vi "220225-VNA RP FLAT.vi"() -> ()   [LabVIEW 2021]
uses:
  Channel parameters.ctl
  Spectrum data.ctl
  vna settings.ctl
  Resonnance detection.ctl
  b7fd31b3-4c8f-4ae8-a038-7c142e2eb182.vi
  <vilib>/Analysis/baseanly.llb/Mean (DBL).vi
  <vilib>/Utility/file.llb/Write Delimited Spreadsheet (DBL).vi
  <vilib>/Comparison/Equal/Equal Functor/Equal Functor.lvclass
  <vilib>/Analysis/NI_AALBase.lvlib
panel:
  in  "RP VNA SETTING":T1={"F start"=200000, "F stop"=2000500, "Sweep size"=1000, "Decimation"=5000, "F_corr"=0, "Ph_OUT1"=0, "Ph_OUT2"=0, "OUT_Lvl1"=32700, "OUT_Lvl2"=32700, "GPIO"=0}
  in  "Amplitude(1V)":dbl=0.3 format="%#_13g"
  out "RP CONNECT":bool
  in  "VOA Calibration cluster":cluster{"PUMP":dbl[], "PROBE":dbl[]}
  out "TRACK DATA REL NO SMOOTHING":dbl[][](array[numeric])
  out "TRACK DATA ABS NO SMOOTHING":dbl[][](array[numeric])
  in  "BTN SAVE TRACK":bool
  in  "BTN STOP TRACK":bool
  out "TRACK REPOSITERY":path
  out "TRACK DATA REL":dbl[][](array[numeric])
  out "TRACK DATA ABS":dbl[][](array[numeric])
  out "Track File List":path[](array[path])
  out "Track Repositery List":path[](array[path])
  out "CHANNEL CHOSEN":i32
  in  "TRACK-STOP":bool
  out "STATUS":string="STOP"
  out "track data":dbl[](array[numeric])=[495490.5081042979, 495481.56129759253, 495478.2328599854, 495479.84884744807, 495476.377462383, 495478.7819904735]
  out "MAIN TAB":T2(tab)
  out "ACQ Indicator":bool
  in  "PUMP":dbl(slide)=100.0 min=0.0 max=100.0 step=0.1 scale=0.0..100.0
  in  "PROBE":dbl(slide)=100.0 min=0.0 max=100.0 step=0.1 scale=0.0..100.0
  in  "BTN RESET VNA":bool
  in  "SPAN":dbl=1900.0 format="%#5.1f"
  in  "STOP":dbl=2000.0 format="%#5.1f"
  in  "CENTER":dbl=1050.0 format="%#5.1f"
  in  "BTN AF VNA":bool
  out "MAGNITUDE/PHASE":cluster{cluster{dbl, dbl}[]}[](graph)
  in  "CHANNEL CHOICE VNA":T3(radio)
  in  "BTN Center to max":bool
  in  "BTN ZOOM-":bool
  in  "BTN ZOOM+":bool
  in  "START":dbl=200.0 format="%#5.1f"
  out "SPACING":dbl=1900.0 min=0.0 max=100.0 step=0.5 format="%#5.1f"
  in  "Points N°":i32=1000 min=600 max=5000 step=1 format="%#4.4g"
  in  "BTN LOOP VNA":bool
  in  "BTN RUN VNA":bool
  in  "BTN SAVE VNA":bool
  in  "BTN FIT DISPLAY":bool caption="FIT DISPLAY"
  in  "BTN AUTOSCALE":bool caption="AUTOSCALE"
  in  "BTN DISPLAY TYPE":bool caption="DISPLAY"
  in  "BTN VIEW PERSISTANCE":bool
  in  "Hide/Show track data channel":bool[](array[boolean])
  in  "BTN AUTOSAVE RAW DATA":bool=TRUE
  in  "COMMENTS":string
  in  "ASSAY NAME":string
  in  "DELAY AFTER SWITCH (s)":i32
  in  "N°POINTS TO DISPLAY":i32=200
  in  "DISPLAY OPTION":u16(ring) items=["Absolute frequency", "Relative frequency (ppm)"]
  in  "DELAY BETWEEN TRIG (s)":i32
  in  "AVERAGE/POINT":dbl=1.0
  out "LIVE TRACK":dbl[][](graph)
  out "CHANNELS IND TRACK":T3(radio)
  in  "BTN RUN TRACK":bool
  in  "TEMPORAL SMOOTHING":i32=15
  in  "BTN NEW TRACK":bool
  in  "BTN PAUSE TRACK":bool
  in  "CHANNELS PARAMETERS":T4[](array[typedef])=[{"START 2"=200.0, "STOP 2"=2000.5, "CENTER 2"=1050.0, "SPAN 2"=1800.0, "CHANNEL TRACK ?"=FALSE, "PUMP"=100.0, "PROBE"=100.0, "Points N° 2"=1000, "SPACING 2"=100.0}, {"START 2"=200.0, "STOP 2"=2000.0, "CENTER 2"=1100.0, "SPAN 2"=1800.0, "CHANNEL TRACK ?"=FALSE, "PUMP"=100.0, "PROBE"=100.0, "Points N° 2"=1000, "SPACING 2"=1800.0}, {"START 2"=200.0, "STOP 2"=2000.0, "CENTER 2"=1100.0, "SPAN 2"=1800.0, "CHANNEL TRACK ?"=FALSE, "PUMP"=100.0, "PROBE"=100.0, "Points N° 2"=1000, "SPACING 2"=1800.0}, {"START 2"=200.0, "STOP 2"=2000.0, "CENTER 2"=1100.0, "SPAN 2"=1800.0, "CHANNEL TRACK ?"=FALSE, "PUMP"=100.0, "PROBE"=100.0, "Points N° 2"=1000, "SPACING 2"=1800.0}, {"START 2"=200.0, "STOP 2"=2000.0, "CENTER 2"=1100.0, "SPAN 2"=1800.0, "CHANNEL TRACK ?"=FALSE, "PUMP"=100.0, "PROBE"=100.0, "Points N° 2"=1000, "SPACING 2"=1800.0}, {"START 2"=200.0, "STOP 2"=2000.0, "CENTER 2"=1100.0, "SPAN 2"=1800.0, "CHANNEL TRACK ?"=FALSE, "PUMP"=100.0, "PROBE"=100.0, "Points N° 2"=1000, "SPACING 2"=1800.0}, {"START 2"=200.0, "STOP 2"=2000.0, "CENTER 2"=1100.0, "SPAN 2"=1800.0, "CHANNEL TRACK ?"=FALSE, "PUMP"=100.0, "PROBE"=100.0, "Points N° 2"=1000, "SPACING 2"=1800.0}, {"START 2"=200.0, "STOP 2"=2000.0, "CENTER 2"=1100.0, "SPAN 2"=1800.0, "CHANNEL TRACK ?"=FALSE, "PUMP"=100.0, "PROBE"=100.0, "Points N° 2"=1000, "SPACING 2"=1800.0}, {"START 2"=200.0, "STOP 2"=2000.0, "CENTER 2"=1100.0, "SPAN 2"=1800.0, "CHANNEL TRACK ?"=FALSE, "PUMP"=100.0, "PROBE"=100.0, "Points N° 2"=1000, "SPACING 2"=1800.0}, {"START 2"=200.0, "STOP 2"=2000.0, "CENTER 2"=1100.0, "SPAN 2"=1800.0, "CHANNEL TRACK ?"=FALSE, "PUMP"=100.0, "PROBE"=100.0, "Points N° 2"=1000, "SPACING 2"=1800.0}, {"START 2"=200.0, "STOP 2"=2000.0, "CENTER 2"=1100.0, "SPAN 2"=1800.0, "CHANNEL TRACK ?"=FALSE, "PUMP"=100.0, "PROBE"=100.0, "Points N° 2"=1000, "SPACING 2"=1800.0}, {"START 2"=200.0, "STOP 2"=2000.0, "CENTER 2"=1100.0, "SPAN 2"=1800.0, "CHANNEL TRACK ?"=FALSE, "PUMP"=100.0, "PROBE"=100.0, "Points N° 2"=1000, "SPACING 2"=1800.0}, {"START 2"=200.0, "STOP 2"=2000.0, "CENTER 2"=1100.0, "SPAN 2"=1800.0, "CHANNEL TRACK ?"=FALSE, "PUMP"=100.0, "PROBE"=100.0, "Points N° 2"=1000, "SPACING 2"=1800.0}, {"START 2"=200.0, "STOP 2"=2000.0, "CENTER 2"=1100.0, "SPAN 2"=1800.0, "CHANNEL TRACK ?"=FALSE, "PUMP"=100.0, "PROBE"=100.0, "Points N° 2"=1000, "SPACING 2"=1800.0}, {"START 2"=200.0, "STOP 2"=2000.0, "CENTER 2"=1100.0, "SPAN 2"=1800.0, "CHANNEL TRACK ?"=FALSE, "PUMP"=100.0, "PROBE"=100.0, "Points N° 2"=1000, "SPACING 2"=1800.0}, {"START 2"=200.0, "STOP 2"=2000.0, "CENTER 2"=1100.0, "SPAN 2"=1800.0, "CHANNEL TRACK ?"=FALSE, "PUMP"=100.0, "PROBE"=100.0, "Points N° 2"=1000, "SPACING 2"=1800.0}] {"SPACING 2" min=0.0 max=100.0 step=0.5; "Points N° 2" min=0 max=100 step=1; "PROBE" min=0.0 max=100.0 step=0.5; "PUMP" min=0.0 max=100.0 step=0.5}
  out "CHANNEL IND SETTINGS":T5(radio)
  in  "RESONNANCE DETECTION":T6={"METHOD"=0, "Parabolic fit"={"Span type"=0, "Fit span"=100.0}} {"Parabolic fit"."Span type" items=["Points N°", "Frequency (Hz)", "Span %"]; "METHOD" items=["Maximum amplitude", "Max on parabolic fit"]}
  in  "TRACK DATA PARAMETERS":cluster{"MAIN FOLDER":path}={"MAIN FOLDER"=path "C:/SensWay Data"}
  in  "SPECTRUM POST PROCESSING PARAMETERS":cluster{"N° SMOOTHING POINTS":i32}={"N° SMOOTHING POINTS"=50}
  in  "AUTOFOCUS PARAMETERS":cluster{"ITERATIONS":i32}={"ITERATIONS"=5}
  in  "CHANNELS":T7
  in  "NETWORK PARAMETERS":T8={"RP-IP 1"="192.168.0.3", "RP-IP 2"="192.168.0.4", "RP-MAC 1"="", "RP-MAC 2"=""}
  in  "VNA DATA CLUSTER":T9
  in  "TRACK DATA CLUSTER":cluster{"CHANNEL":dbl, "KPI 1 TRACK":ext[]}
  out "LOOP ACT":bool
  out "RAW Freq table":dbl[](array[numeric])=[200000.0, 201802.3023023023, 203604.6046046046, 205406.9069069069, 207209.20920920922, 209011.51151151152, 210813.81381381382, 212616.1161161161, 214418.4184184184, 216220.7207207207, 218023.02302302304, 219825.32532532534, 221627.62762762763, 223429.92992992993, 225232.23223223223, 227034.53453453453, 228836.83683683682, 230639.13913913915, 232441.44144144145, 234243.74374374375, 236046.04604604605, 237848.34834834834, 239650.65065065064, 241452.95295295294, 243255.25525525527, 245057.55755755756, 246859.85985985986, 248662.16216216216, 250464.46446446446, 252266.76676676676, 254069.06906906905, 255871.37137137138, 257673.67367367368, 259475.97597597598, 261278.27827827827, 263080.5805805806, 264882.8828828829, 266685.18518518517, 268487.4874874875, 270289.7897897898, 272092.0920920921, 273894.39439439436, 275696.6966966967, 277498.998998999, 279301.3013013013, 281103.6036036036, 282905.9059059059, 284708.2082082082, 286510.51051051053, 288312.8128128128, 290115.1151151151, 291917.4174174174, 293719.7197197197, 295522.02202202205, 297324.3243243243, 299126.6266266266, 300928.9289289289, 302731.23123123124, 304533.5335335335, 306335.83583583584, 308138.1381381381, 309940.44044044043, 311742.74274274276, 313545.04504504503, 315347.34734734736, 317149.6496496496, 318951.95195195195, 320754.2542542543, 322556.55655655655, 324358.8588588588, 326161.16116116114, 327963.4634634635, 329765.76576576574, 331568.06806806807, 333370.37037037034, 335172.67267267266, 336974.974974975, 338777.27727727726, 340579.5795795796, 342381.88188188185, 344184.1841841842, 345986.4864864865, 347788.7887887888, 349591.09109109105, 351393.3933933934, 353195.6956956957, 354997.997997998, 356800.3003003003, 358602.60260260256, 360404.9049049049, 362207.2072072072, 364009.50950950955, 365811.8118118118, 367614.1141141141, 369416.4164164164, 371218.71871871874, 373021.021021021, 374823.3233233233, 376625.6256256256, 378427.9279279279, 380230.23023023026, 382032.5325325325, 383834.8348348348, 385637.1371371371, 387439.43943943945, 389241.7417417418, 391044.04404404404, 392846.3463463463, 394648.64864864864, 396450.95095095097, 398253.25325325324, 400055.5555555555, 401857.85785785783, 403660.16016016016, 405462.4624624625, 407264.76476476475, 409067.067067067, 410869.36936936935, 412671.6716716717, 414473.973973974, 416276.2762762763, 418078.57857857854, 419880.88088088087, 421683.1831831832, 423485.48548548546, 425287.7877877878, 427090.09009009006, 428892.3923923924, 430694.6946946947, 432496.996996997, 434299.29929929925, 436101.6016016016, 437903.9039039039, 439706.20620620623, 441508.5085085085, 443310.81081081077, 445113.1131131131, 446915.4154154154, 448717.7177177177, 450520.02002002, 452322.3223223223, 454124.6246246246, 455926.92692692694, 457729.2292292292, 459531.5315315315, 461333.8338338338, 463136.13613613613, 464938.4384384384, 466740.74074074073, 468543.04304304306, 470345.3453453453, 472147.64764764765, 473949.9499499499, 475752.25225225225, 477554.5545545545, 479356.85685685684, 481159.1591591592, 482961.46146146144, 484763.76376376377, 486566.06606606604, 488368.36836836836, 490170.67067067063, 491972.97297297296, 493775.2752752753, 495577.57757757755, 497379.8798798799, 499182.18218218215, 500984.4844844845, 502786.78678678675, 504589.0890890891, 506391.3913913914, 508193.69369369367, 509995.995995996, 511798.29829829826, 513600.6006006006, 515402.90290290286, 517205.2052052052, 519007.5075075075, 520809.8098098098, 522612.1121121121, 524414.4144144144, 526216.7167167168, 528019.0190190191, 529821.3213213213, 531623.6236236236, 533425.9259259258, 535228.2282282282, 537030.5305305305, 538832.8328328328, 540635.1351351351, 542437.4374374375, 544239.7397397398, 546042.042042042, 547844.3443443443, 549646.6466466465, 551448.9489489489, 553251.2512512512, 555053.5535535535, 556855.8558558559, 558658.1581581582, 560460.4604604605, 562262.7627627627, 564065.065065065, 565867.3673673674, 567669.6696696696, 569471.9719719719, 571274.2742742742, 573076.5765765766, 574878.8788788789, 576681.1811811812, 578483.4834834835, 580285.7857857858, 582088.0880880881, 583890.3903903903, 585692.6926926926, 587494.994994995, 589297.2972972973, 591099.5995995996, 592901.9019019019, 594704.2042042043, 596506.5065065065, 598308.8088088088, 600111.111111111, 601913.4134134133, 603715.7157157157, 605518.018018018, 607320.3203203203, 609122.6226226226, 610924.924924925, 612727.2272272272, 614529.5295295295, 616331.8318318318, 618134.134134134, 619936.4364364364, 621738.7387387387, 623541.041041041, 625343.3433433434, 627145.6456456457, 628947.947947948, 630750.2502502502, 632552.5525525525, 634354.8548548548, 636157.1571571571, 637959.4594594594, 639761.7617617617, 641564.0640640641, 643366.3663663664, 645168.6686686687, 646970.9709709709, 648773.2732732733, 650575.5755755756, 652377.8778778778, 654180.1801801801, 655982.4824824824, 657784.7847847848, 659587.0870870871, 661389.3893893894, 663191.6916916918, 664993.993993994, 666796.2962962963, 668598.5985985985, 670400.9009009008, 672203.2032032032, 674005.5055055055, 675807.8078078078, 677610.1101101101, 679412.4124124125, 681214.7147147147, 683017.017017017, 684819.3193193192, 686621.6216216215, 688423.9239239239, 690226.2262262262, 692028.5285285285, 693830.8308308308, 695633.1331331332, 697435.4354354354, 699237.7377377377, 701040.04004004, 702842.3423423423, 704644.6446446446, 706446.9469469469, 708249.2492492492, 710051.5515515516, 711853.8538538539, 713656.1561561562, 715458.4584584584, 717260.7607607607, 719063.063063063, 720865.3653653653, 722667.6676676676, 724469.9699699699, 726272.2722722723, 728074.5745745746, 729876.8768768768, 731679.1791791791, 733481.4814814815, 735283.7837837838, 737086.0860860861, 738888.3883883883, 740690.6906906907, 742492.992992993, 744295.2952952953, 746097.5975975975, 747899.8998998998, 749702.2022022022, 751504.5045045045, 753306.8068068068, 755109.109109109, 756911.4114114114, 758713.7137137137, 760516.016016016, 762318.3183183183, 764120.6206206206, 765922.9229229229, 767725.2252252252, 769527.5275275275, 771329.8298298299, 773132.1321321321, 774934.4344344344, 776736.7367367367, 778539.039039039, 780341.3413413413, 782143.6436436436, 783945.9459459459, 785748.2482482482, 787550.5505505506, 789352.8528528528, 791155.1551551551, 792957.4574574574, 794759.7597597598, 796562.0620620621, 798364.3643643643, 800166.6666666666, 801968.968968969, 803771.2712712713, 805573.5735735735, 807375.8758758758, 809178.1781781781, 810980.4804804805, 812782.7827827828, 814585.085085085, 816387.3873873873, 818189.6896896897, 819991.991991992, 821794.2942942943, 823596.5965965965, 825398.8988988989, 827201.2012012012, 829003.5035035035, 830805.8058058057, 832608.108108108, 834410.4104104104, 836212.7127127127, 838015.015015015, 839817.3173173172, 841619.6196196196, 843421.9219219219, 845224.2242242242, 847026.5265265265, 848828.8288288288, 850631.1311311311, 852433.4334334334, 854235.7357357357, 856038.0380380381, 857840.3403403403, 859642.6426426426, 861444.9449449449, 863247.2472472473, 865049.5495495495, 866851.8518518518, 868654.1541541541, 870456.4564564564, 872258.7587587588, 874061.061061061, 875863.3633633633, 877665.6656656656, 879467.967967968, 881270.2702702703, 883072.5725725725, 884874.8748748748, 886677.1771771772, 888479.4794794795, 890281.7817817817, 892084.084084084, 893886.3863863864, 895688.6886886887, 897490.990990991, 899293.2932932932, 901095.5955955955, 902897.8978978979, 904700.2002002002, 906502.5025025025, 908304.8048048047, 910107.1071071071, 911909.4094094094, 913711.7117117117, 915514.0140140139, 917316.3163163163, 919118.6186186186, 920920.9209209209, 922723.2232232232, 924525.5255255254, 926327.8278278278, 928130.1301301301, 929932.4324324324, 931734.7347347348, 933537.037037037, 935339.3393393393, 937141.6416416416, 938943.943943944, 940746.2462462463, 942548.5485485485, 944350.8508508508, 946153.1531531531, 947955.4554554555, 949757.7577577577, 951560.06006006, 953362.3623623623, 955164.6646646647, 956966.966966967, 958769.2692692692, 960571.5715715715, 962373.8738738738, 964176.1761761762, 965978.4784784785, 967780.7807807807, 969583.083083083, 971385.3853853854, 973187.6876876877, 974989.9899899899, 976792.2922922922, 978594.5945945946, 980396.8968968969, 982199.1991991992, 984001.5015015014, 985803.8038038037, 987606.1061061061, 989408.4084084084, 991210.7107107107, 993013.0130130129, 994815.3153153153, 996617.6176176176, 998419.9199199199, 1000222.2222222221, 1002024.5245245245, 1003826.8268268268, 1005629.1291291291, 1007431.4314314314, 1009233.7337337337, 1011036.036036036, 1012838.3383383383, 1014640.6406406406, 1016442.942942943, 1018245.2452452452, 1020047.5475475475, 1021849.8498498498, 1023652.1521521521, 1025454.4544544544, 1027256.7567567567, 1029059.059059059, 1030861.3613613613, 1032663.6636636637, 1034465.9659659659, 1036268.2682682682, 1038070.5705705705, 1039872.8728728729, 1041675.1751751752, 1043477.4774774774, 1045279.7797797797, 1047082.082082082, 1048884.3843843844, 1050686.6866866867, 1052488.988988989, 1054291.2912912914, 1056093.5935935937, 1057895.895895896, 1059698.198198198, 1061500.5005005004, 1063302.8028028028, 1065105.105105105, 1066907.4074074074, 1068709.7097097095, 1070512.0120120118, 1072314.3143143142, 1074116.6166166165, 1075918.9189189188, 1077721.2212212211, 1079523.5235235235, 1081325.8258258258, 1083128.1281281281, 1084930.4304304305, 1086732.7327327328, 1088535.035035035, 1090337.3373373374, 1092139.6396396398, 1093941.9419419419, 1095744.2442442442, 1097546.5465465465, 1099348.8488488488, 1101151.1511511512, 1102953.4534534533, 1104755.7557557556, 1106558.058058058, 1108360.3603603602, 1110162.6626626626, 1111964.964964965, 1113767.2672672672, 1115569.5695695695, 1117371.8718718719, 1119174.1741741742, 1120976.4764764765, 1122778.7787787789, 1124581.0810810812, 1126383.3833833835, 1128185.6856856856, 1129987.987987988, 1131790.2902902903, 1133592.5925925926, 1135394.894894895, 1137197.197197197, 1138999.4994994993, 1140801.8018018017, 1142604.104104104, 1144406.4064064063, 1146208.7087087086, 1148011.011011011, 1149813.3133133133, 1151615.6156156156, 1153417.917917918, 1155220.2202202203, 1157022.5225225226, 1158824.824824825, 1160627.1271271273, 1162429.4294294294, 1164231.7317317317, 1166034.034034034, 1167836.3363363363, 1169638.6386386384, 1171440.9409409408, 1173243.243243243, 1175045.5455455454, 1176847.8478478477, 1178650.15015015, 1180452.4524524524, 1182254.7547547547, 1184057.057057057, 1185859.3593593594, 1187661.6616616617, 1189463.963963964, 1191266.2662662663, 1193068.5685685687, 1194870.8708708708, 1196673.173173173, 1198475.4754754754, 1200277.7777777778, 1202080.08008008, 1203882.3823823822, 1205684.6846846845, 1207486.9869869868, 1209289.2892892892, 1211091.5915915915, 1212893.8938938938, 1214696.1961961961, 1216498.4984984985, 1218300.8008008008, 1220103.103103103, 1221905.4054054054, 1223707.7077077078, 1225510.01001001, 1227312.3123123124, 1229114.6146146145, 1230916.9169169168, 1232719.2192192192, 1234521.5215215215, 1236323.8238238238, 1238126.126126126, 1239928.4284284282, 1241730.7307307306, 1243533.033033033, 1245335.3353353352, 1247137.6376376376, 1248939.9399399399, 1250742.2422422422, 1252544.5445445445, 1254346.8468468469, 1256149.1491491492, 1257951.4514514515, 1259753.7537537536, 1261556.056056056, 1263358.3583583583, 1265160.6606606606, 1266962.962962963, 1268765.2652652652, 1270567.5675675676, 1272369.86986987, 1274172.1721721722, 1275974.4744744743, 1277776.7767767766, 1279579.079079079, 1281381.3813813813, 1283183.6836836836, 1284985.985985986, 1286788.2882882883, 1288590.5905905906, 1290392.892892893, 1292195.195195195, 1293997.4974974974, 1295799.7997997997, 1297602.102102102, 1299404.4044044043, 1301206.7067067067, 1303009.009009009, 1304811.3113113113, 1306613.6136136136, 1308415.915915916, 1310218.218218218, 1312020.5205205204, 1313822.8228228227, 1315625.125125125, 1317427.4274274274, 1319229.7297297297, 1321032.032032032, 1322834.3343343344, 1324636.6366366367, 1326438.9389389388, 1328241.241241241, 1330043.5435435434, 1331845.8458458458, 1333648.148148148, 1335450.4504504504, 1337252.7527527527, 1339055.055055055, 1340857.3573573574, 1342659.6596596597, 1344461.9619619618, 1346264.2642642641, 1348066.5665665665, 1349868.8688688688, 1351671.1711711711, 1353473.4734734735, 1355275.7757757758, 1357078.078078078, 1358880.3803803804, 1360682.6826826825, 1362484.9849849849, 1364287.2872872872, 1366089.5895895895, 1367891.8918918918, 1369694.1941941942, 1371496.4964964965, 1373298.7987987988, 1375101.1011011011, 1376903.4034034032, 1378705.7057057056, 1380508.008008008, 1382310.3103103102, 1384112.6126126125, 1385914.9149149149, 1387717.2172172172, 1389519.5195195195, 1391321.8218218219, 1393124.1241241242, 1394926.4264264263, 1396728.7287287286, 1398531.031031031, 1400333.3333333333, 1402135.6356356356, 1403937.937937938, 1405740.2402402402, 1407542.5425425426, 1409344.844844845, 1411147.147147147, 1412949.4494494493, 1414751.7517517516, 1416554.054054054, 1418356.3563563563, 1420158.6586586586, 1421960.960960961, 1423763.2632632633, 1425565.5655655656, 1427367.867867868, 1429170.17017017, 1430972.4724724723, 1432774.7747747747, 1434577.077077077, 1436379.3793793793, 1438181.6816816817, 1439983.983983984, 1441786.2862862863, 1443588.5885885886, 1445390.8908908907, 1447193.193193193, 1448995.4954954954, 1450797.7977977977, 1452600.1001001, 1454402.4024024024, 1456204.7047047047, 1458007.007007007, 1459809.3093093093, 1461611.6116116114, 1463413.9139139138, 1465216.216216216, 1467018.5185185184, 1468820.8208208208, 1470623.123123123, 1472425.4254254254, 1474227.7277277277, 1476030.03003003, 1477832.3323323324, 1479634.6346346345, 1481436.9369369368, 1483239.2392392391, 1485041.5415415415, 1486843.8438438438, 1488646.146146146, 1490448.4484484484, 1492250.7507507508, 1494053.053053053, 1495855.3553553552, 1497657.6576576575, 1499459.9599599598, 1501262.2622622622, 1503064.5645645645, 1504866.8668668668, 1506669.1691691692, 1508471.4714714715, 1510273.7737737738, 1512076.0760760761, 1513878.3783783782, 1515680.6806806806, 1517482.9829829829, 1519285.2852852852, 1521087.5875875875, 1522889.8898898899, 1524692.1921921922, 1526494.4944944945, 1528296.7967967968, 1530099.099099099, 1531901.4014014013, 1533703.7037037036, 1535506.006006006, 1537308.3083083082, 1539110.6106106106, 1540912.912912913, 1542715.2152152152, 1544517.5175175176, 1546319.8198198196, 1548122.122122122, 1549924.4244244243, 1551726.7267267266, 1553529.029029029, 1555331.3313313313, 1557133.6336336336, 1558935.935935936, 1560738.2382382383, 1562540.5405405406, 1564342.8428428427, 1566145.145145145, 1567947.4474474473, 1569749.7497497497, 1571552.052052052, 1573354.3543543543, 1575156.6566566566, 1576958.958958959, 1578761.2612612613, 1580563.5635635634, 1582365.8658658657, 1584168.168168168, 1585970.4704704704, 1587772.7727727727, 1589575.075075075, 1591377.3773773774, 1593179.6796796797, 1594981.981981982, 1596784.2842842843, 1598586.5865865864, 1600388.8888888888, 1602191.191191191, 1603993.4934934934, 1605795.7957957957, 1607598.098098098, 1609400.4004004004, 1611202.7027027027, 1613005.005005005, 1614807.3073073071, 1616609.6096096095, 1618411.9119119118, 1620214.2142142141, 1622016.5165165165, 1623818.8188188188, 1625621.121121121, 1627423.4234234234, 1629225.7257257258, 1631028.0280280279, 1632830.3303303302, 1634632.6326326325, 1636434.9349349348, 1638237.2372372372, 1640039.5395395395, 1641841.8418418418, 1643644.1441441441, 1645446.4464464465, 1647248.7487487488, 1649051.051051051, 1650853.3533533532, 1652655.6556556555, 1654457.9579579579, 1656260.2602602602, 1658062.5625625625, 1659864.8648648649, 1661667.1671671672, 1663469.4694694695, 1665271.7717717716, 1667074.074074074, 1668876.3763763763, 1670678.6786786786, 1672480.980980981, 1674283.2832832832, 1676085.5855855856, 1677887.887887888, 1679690.1901901902, 1681492.4924924925, 1683294.7947947946, 1685097.097097097, 1686899.3993993993, 1688701.7017017016, 1690504.004004004, 1692306.3063063063, 1694108.6086086086, 1695910.910910911, 1697713.2132132133, 1699515.5155155153, 1701317.8178178177, 1703120.12012012, 1704922.4224224223, 1706724.7247247247, 1708527.027027027, 1710329.3293293293, 1712131.6316316316, 1713933.933933934, 1715736.236236236, 1717538.5385385384, 1719340.8408408407, 1721143.143143143, 1722945.4454454454, 1724747.7477477477, 1726550.05005005, 1728352.3523523523, 1730154.6546546547, 1731956.956956957, 1733759.259259259, 1735561.5615615614, 1737363.8638638637, 1739166.166166166, 1740968.4684684684, 1742770.7707707707, 1744573.073073073, 1746375.3753753754, 1748177.6776776777, 1749979.9799799798, 1751782.2822822821, 1753584.5845845845, 1755386.8868868868, 1757189.189189189, 1758991.4914914914, 1760793.7937937938, 1762596.096096096, 1764398.3983983984, 1766200.7007007005, 1768003.0030030028, 1769805.3053053052, 1771607.6076076075, 1773409.9099099098, 1775212.2122122122, 1777014.5145145145, 1778816.8168168168, 1780619.1191191191, 1782421.4214214215, 1784223.7237237236, 1786026.0260260259, 1787828.3283283282, 1789630.6306306305, 1791432.9329329329, 1793235.2352352352, 1795037.5375375375, 1796839.8398398398, 1798642.1421421422, 1800444.4444444443, 1802246.7467467466, 1804049.049049049, 1805851.3513513512, 1807653.6536536536, 1809455.955955956, 1811258.2582582582, 1813060.5605605606, 1814862.8628628629, 1816665.1651651652, 1818467.4674674673, 1820269.7697697696, 1822072.072072072, 1823874.3743743743, 1825676.6766766766, 1827478.978978979, 1829281.2812812813, 1831083.5835835836, 1832885.885885886, 1834688.188188188, 1836490.4904904903, 1838292.7927927927, 1840095.095095095, 1841897.3973973973, 1843699.6996996996, 1845502.002002002, 1847304.3043043043, 1849106.6066066066, 1850908.9089089087, 1852711.211211211, 1854513.5135135134, 1856315.8158158157, 1858118.118118118, 1859920.4204204204, 1861722.7227227227, 1863525.025025025, 1865327.3273273273, 1867129.6296296297, 1868931.9319319318, 1870734.234234234, 1872536.5365365364, 1874338.8388388387, 1876141.141141141, 1877943.4434434434, 1879745.7457457457, 1881548.048048048, 1883350.3503503504, 1885152.6526526525, 1886954.9549549548, 1888757.2572572571, 1890559.5595595594, 1892361.8618618618, 1894164.164164164, 1895966.4664664664, 1897768.7687687688, 1899571.071071071, 1901373.3733733734, 1903175.6756756755, 1904977.9779779778, 1906780.2802802802, 1908582.5825825825, 1910384.8848848848, 1912187.1871871871, 1913989.4894894895, 1915791.7917917918, 1917594.0940940941, 1919396.3963963962, 1921198.6986986985, 1923001.0010010009, 1924803.3033033032, 1926605.6056056055, 1928407.9079079079, 1930210.2102102102, 1932012.5125125125, 1933814.8148148148, 1935617.117117117, 1937419.4194194193, 1939221.7217217216, 1941024.024024024, 1942826.3263263262, 1944628.6286286286, 1946430.930930931, 1948233.2332332332, 1950035.5355355355, 1951837.8378378379, 1953640.14014014, 1955442.4424424423, 1957244.7447447446, 1959047.047047047, 1960849.3493493493, 1962651.6516516516, 1964453.953953954, 1966256.2562562563, 1968058.5585585586, 1969860.8608608607, 1971663.163163163, 1973465.4654654653, 1975267.7677677677, 1977070.07007007, 1978872.3723723723, 1980674.6746746746, 1982476.976976977, 1984279.2792792793, 1986081.5815815816, 1987883.8838838837, 1989686.186186186, 1991488.4884884884, 1993290.7907907907, 1995093.093093093, 1996895.3953953953, 1998697.6976976977, 2000500.0]
  in  "ENABLE INTERNAL MODULATION":bool=TRUE
  in  "VNA DATA CLUSTER TBL":T9[](array[typedef])
  in  "TRACK DATA CLUSTER TBL":cluster{"CHANNEL":dbl, "KPI 1 TRACK":ext[]}[](array[cluster])
  in  "PERSISTANCE DATA CLUSTER":T9
  in  "VNA SETTING CLUSTER":T4 {"SPACING 2" min=0.0 max=100.0 step=0.5; "Points N° 2" min=0 max=100 step=1; "PROBE" min=0.0 max=100.0 step=0.5; "PUMP" min=0.0 max=100.0 step=0.5}
  out "Information tips":string
  in  "PANEL VNA":bool
  in  "PANEL TRACKING":bool
  in  "BTN STOP":bool
  in  "PANEL GENERAL SETTINGS":bool
  in  "PANEL TRACK SETTINGS":bool
  # "E"
  # "POINTS"
  # "SPACING"
  # "TRACK ?"
  # "START"
  # "STOP"
  # "CENTER"
  # "SPAN"
  # "PROBE"
  # "PUMP"
  # "PARAMETERS"
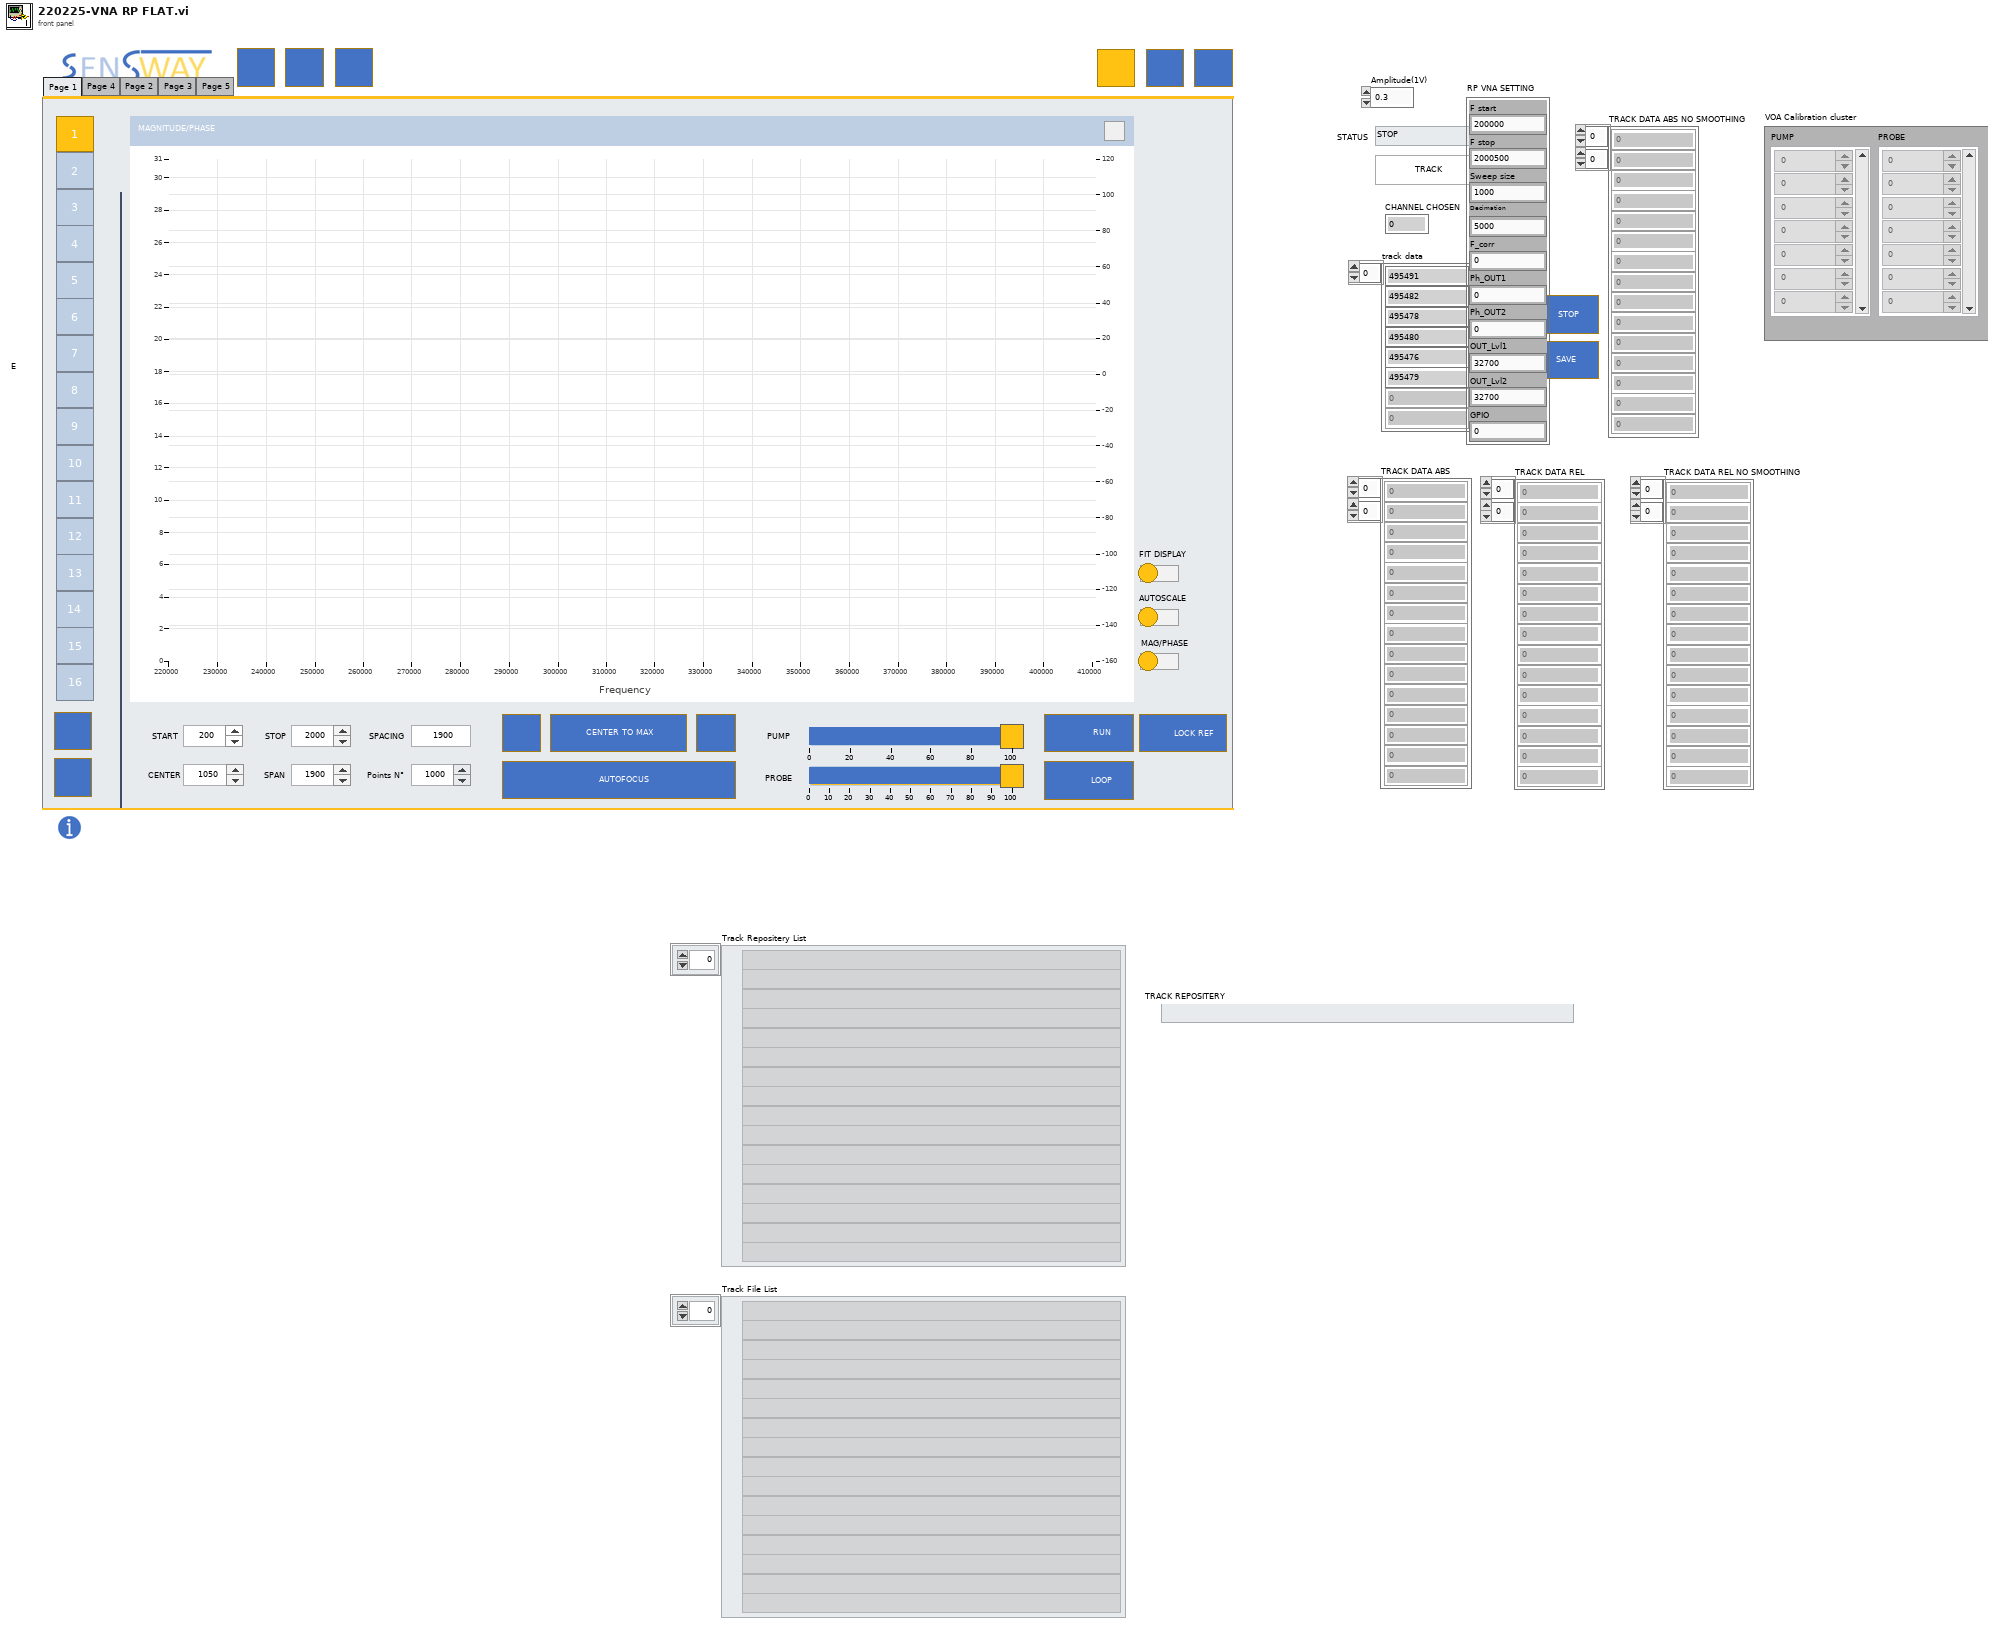
[diagram p1: front panel]
types:
  T1 = typedef "vna settings.ctl" = cluster{"F start":u32, "F stop":u32, "Sweep size":u32, "Decimation":u32, "F_corr":u32, "Ph_OUT1":u32, "Ph_OUT2":u32, "OUT_Lvl1":u32, "OUT_Lvl2":u32, "GPIO":u32}
  T2 = enum32{"Page 1", "Page 4", "Page 2", "Page 3", "Page 5"}
  T3 = enum32{"Button 1", "Button 2", "Button 3", "Sélection radio 4", "Sélection radio 5", "Sélection radio 6", "Sélection radio 7", "Sélection radio 8", "Sélection radio 9", "Sélection radio 10", "Sélection radio 11", "Sélection radio 12", "Sélection radio 13", "Sélection radio 14", "Sélection radio 15", "Sélection radio 16"}
  T4 = typedef "Channel parameters.ctl" = cluster{"START 2":dbl, "STOP 2":dbl, "CENTER 2":dbl, "SPAN 2":dbl, "CHANNEL TRACK ?":bool, "PUMP":dbl, "PROBE":dbl, "Points N° 2":i32, "SPACING 2":dbl}
  T5 = enum32{"No Selection", "Button 1", "Button 2", "Button 3", "Sélection radio 4", "Sélection radio 5", "Sélection radio 6", "Sélection radio 7", "Sélection radio 8", "Sélection radio 9", "Sélection radio 10", "Sélection radio 11", "Sélection radio 12", "Sélection radio 13", "Sélection radio 14", "Sélection radio 15", "Sélection radio 16"}
  T6 = typedef "Resonnance detection.ctl" = cluster{"METHOD":u16, "Parabolic fit":cluster{"Span type":u16, "Fit span":dbl}}
  T7 = cluster{"CHANNEL 1":bool, "CHANNEL 2":bool, "CHANNEL 3":bool, "CHANNEL 4":bool, "CHANNEL 5":bool, "CHANNEL 6":bool, "CHANNEL 7":bool, "CHANNEL 8":bool, "CHANNEL 9":bool, "CHANNEL 10":bool, "CHANNEL 11":bool, "CHANNEL 12":bool, "CHANNEL 13":bool, "CHANNEL 14":bool, "CHANNEL 15":bool, "CHANNEL 16":bool}
  T8 = cluster{"RP-IP 1":string, "RP-IP 2":string, "RP-MAC 1":string, "RP-MAC 2":string}
  T9 = typedef "Spectrum data.ctl" = cluster{"CHANNEL":dbl, "FREQUENCY TABLE":ext[], "MAGNITUDE TABLE":ext[], "PHASE TABLE":ext[], "REAL TABLE":ext[], "IMAGINARY TABLE":ext[]}
  T10 = cluster{"START 2":dbl, "STOP 2":dbl, "CENTER 2":dbl, "SPAN 2":dbl, "CHANNEL TRACK ?":bool, "PUMP":dbl, "PROBE":dbl, "Points N° 2":i32, "SPACING 2":dbl}[]
  T11 = enum16{"Freq start", "Freq stop", "Sweep size", "Decimation rate", "Freq corr", "Phase output 1", "Phase output 2", "Output level 1", "Output level 2", "GPIO", "SWEEP START"}
  T12 = enum8{"Enabled", "Disabled", "Disabled and Grayed Out"}
  T13 = cluster{"FREQUENCY":sgl[], "REAL 1":dbl[], "IMAGINARY 1":sgl[], "MAGNITUDE 1":dbl[], "PHASE 1":dbl[], "REAL 2":dbl[], "IMAGINARY 2":sgl[], "MAGNITUDE 2":dbl[], "PHASE 2":dbl[]}
  T14 = cluster{cluster{"Numeric Control":ext, "Numeric Control":ext}[]}[]
  T15 = cluster{"F start":u32, "F stop":u32, "Sweep size":u32, "Decimation":u32, "F_corr":u32, "Ph_OUT1":u32, "Ph_OUT2":u32, "OUT_Lvl1":u32, "OUT_Lvl2":u32, "GPIO":u32}
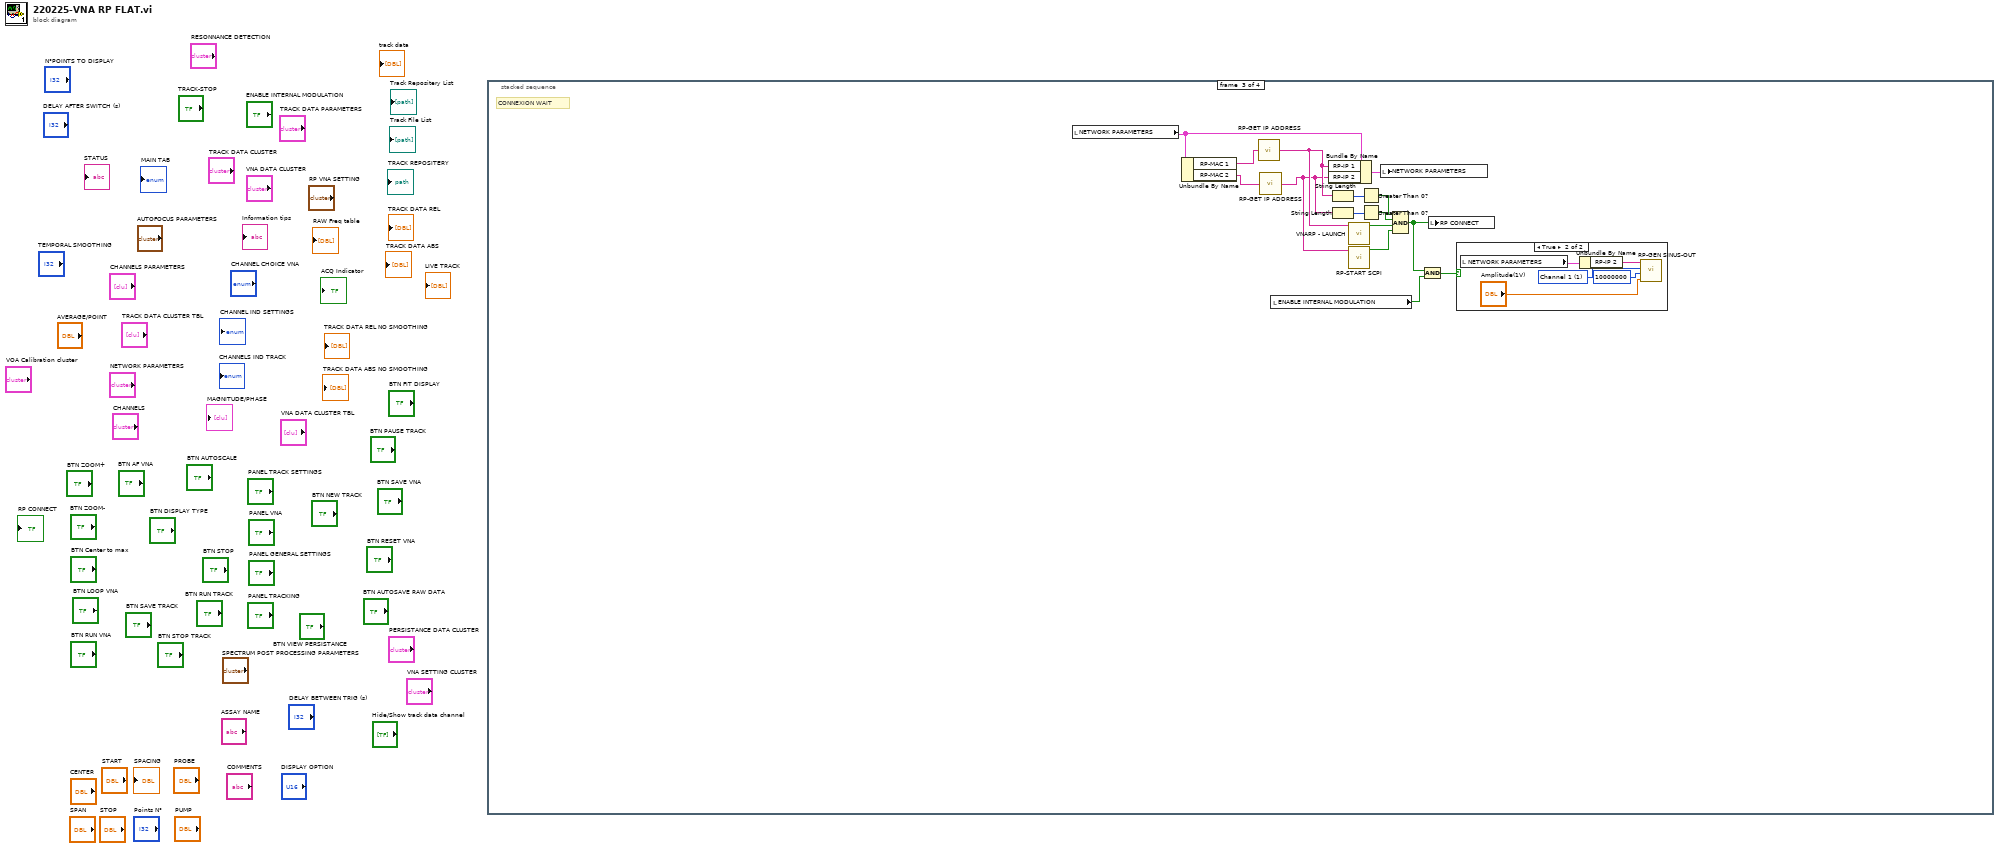
[diagram p0: block diagram]
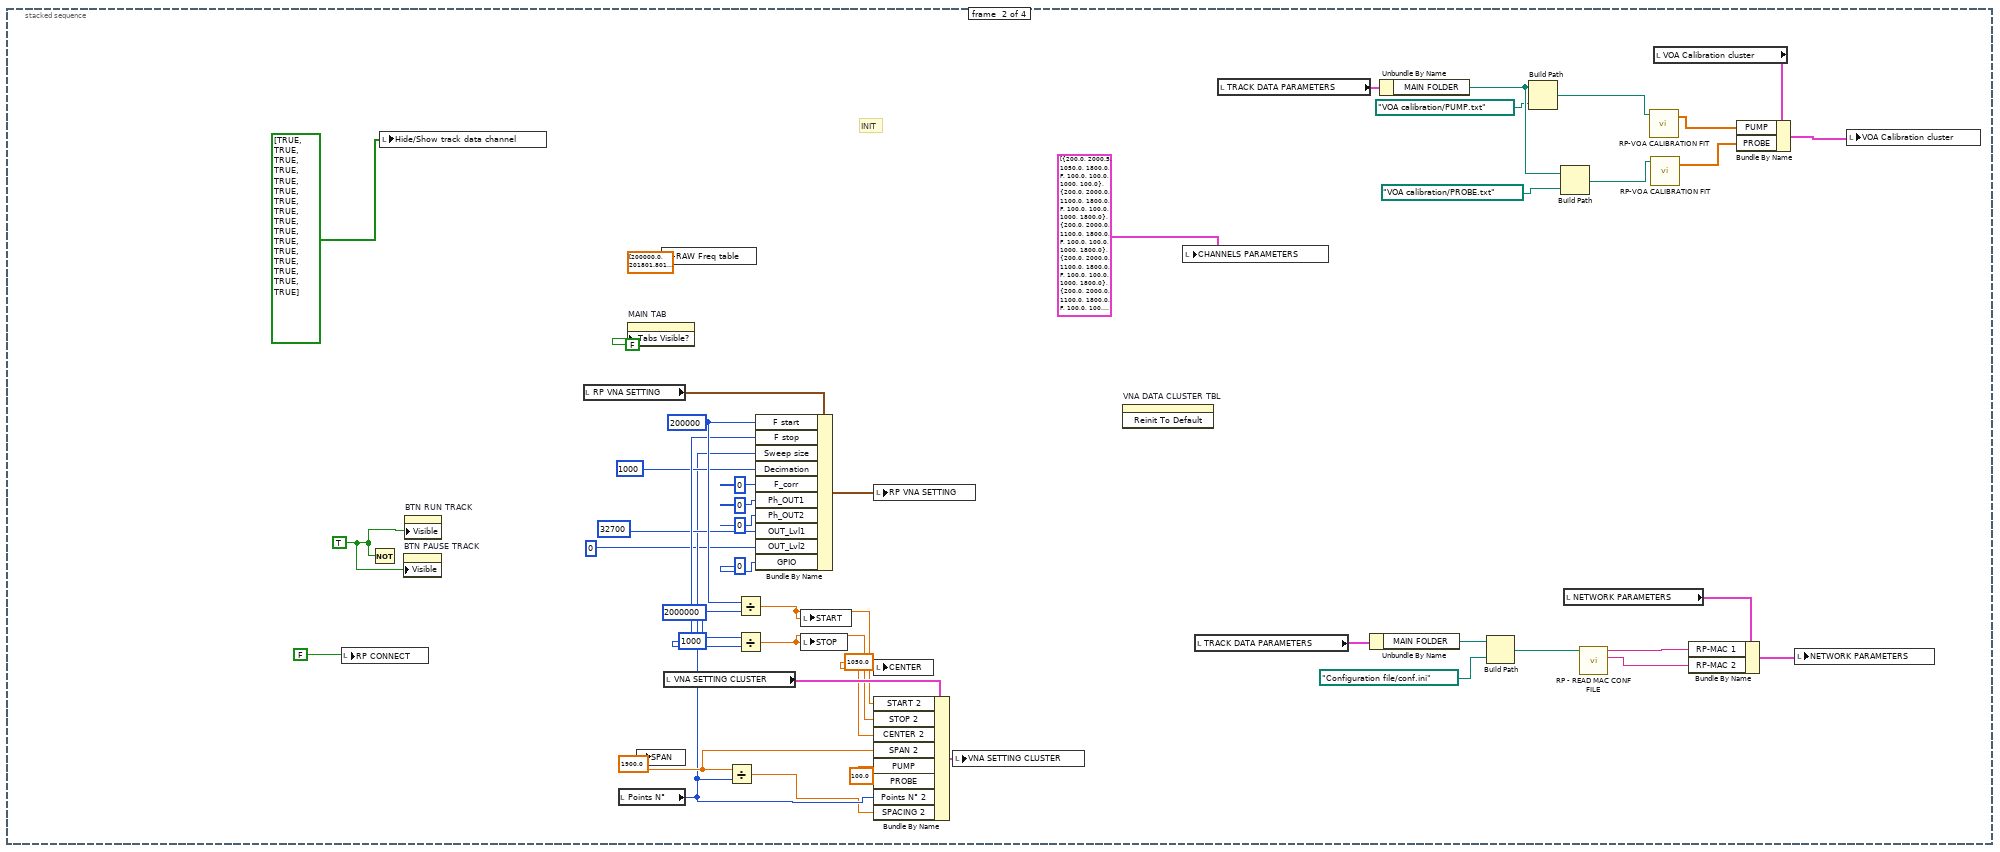
[diagram p3: hidden frame]
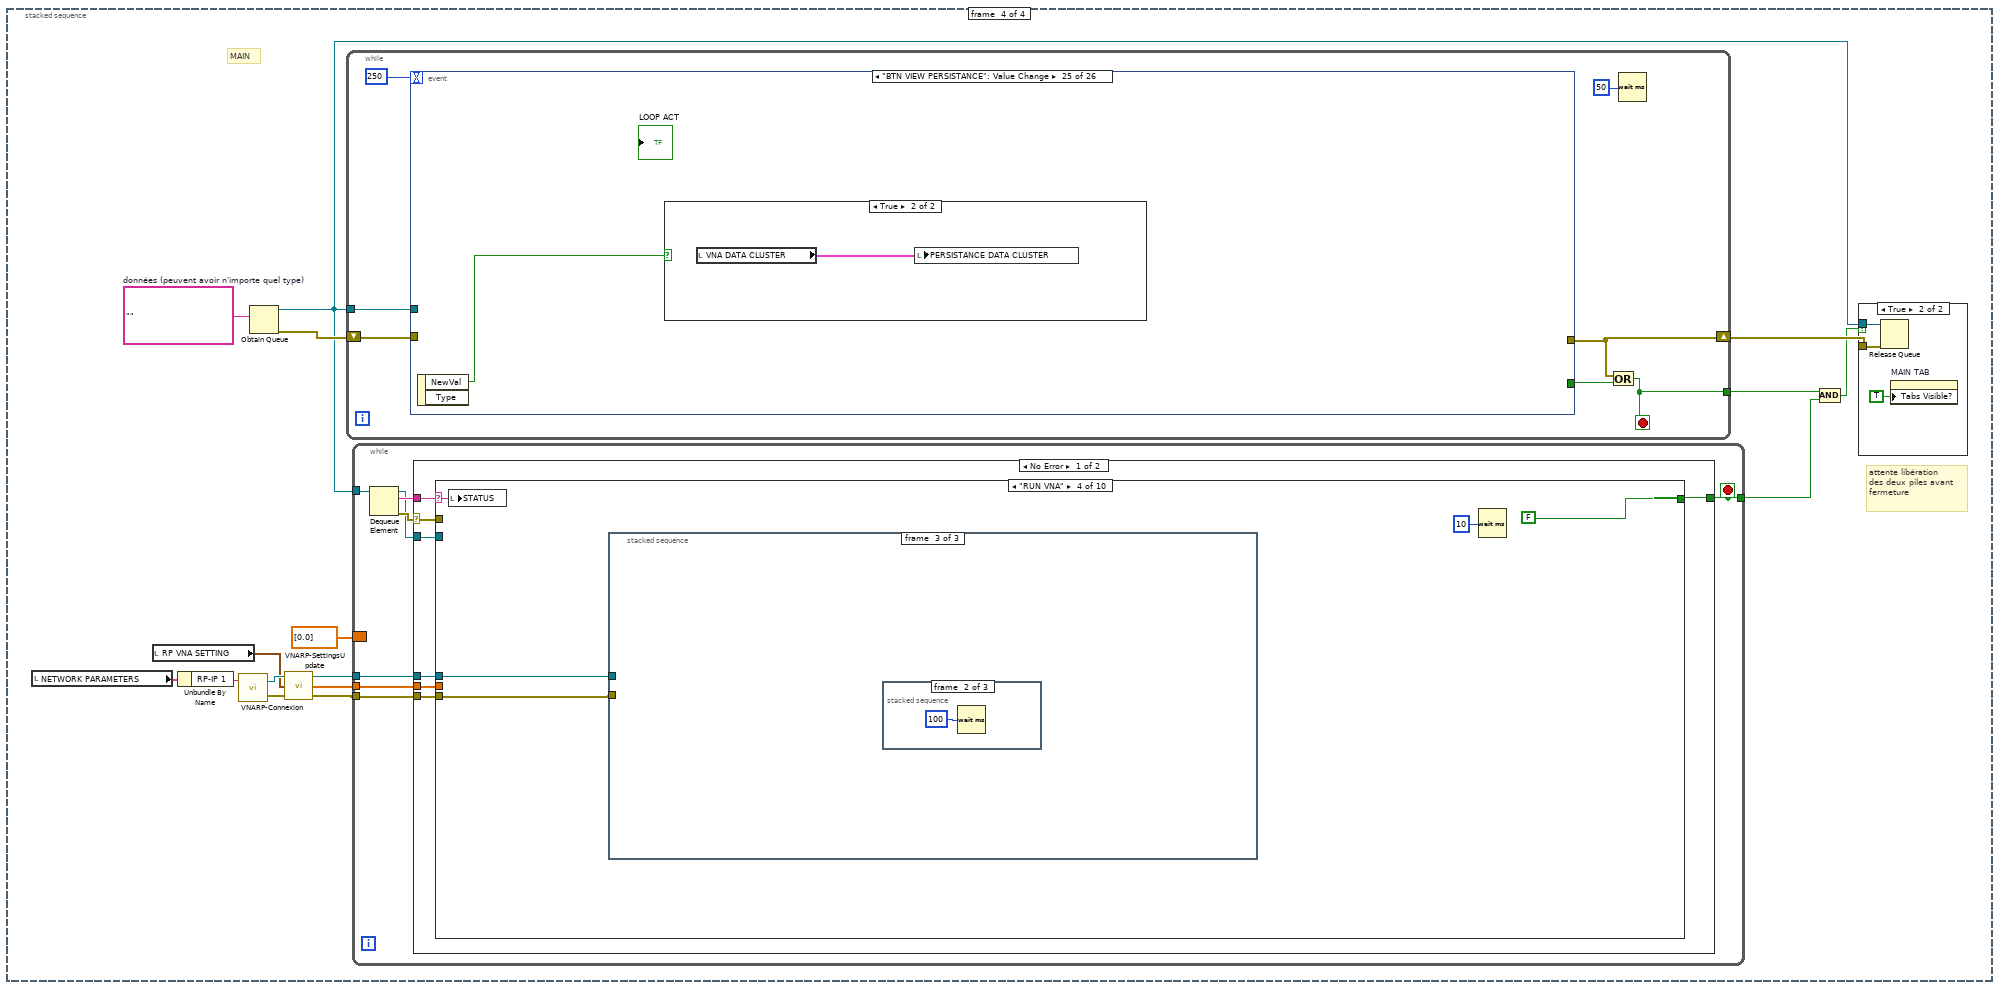
[diagram p5: hidden frame]
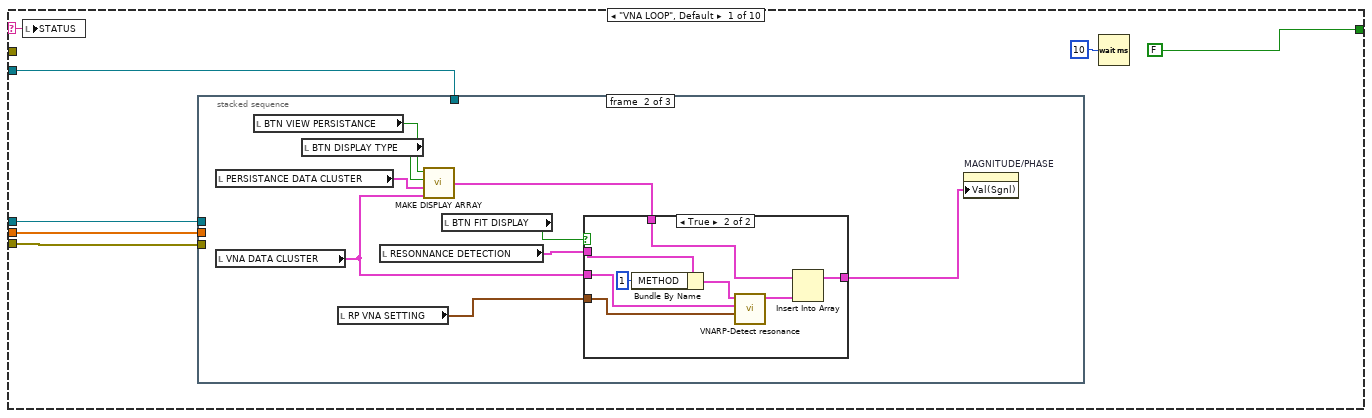
[diagram p7: hidden frame]
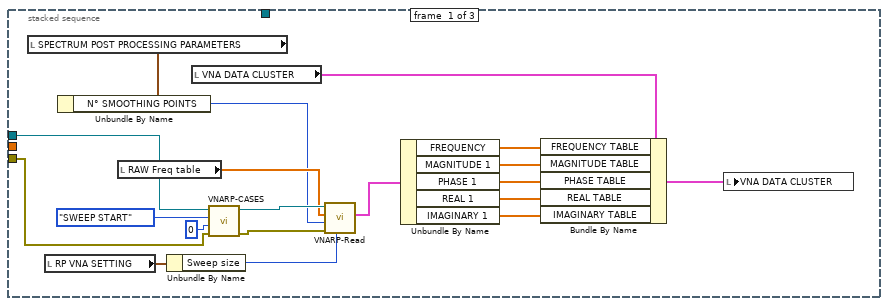
[diagram p8: hidden frame]
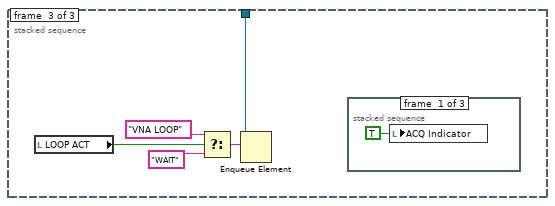
[diagram p10: hidden frame]
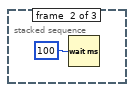
[diagram p11: hidden frame]
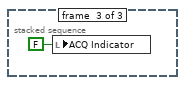
[diagram p12: hidden frame]
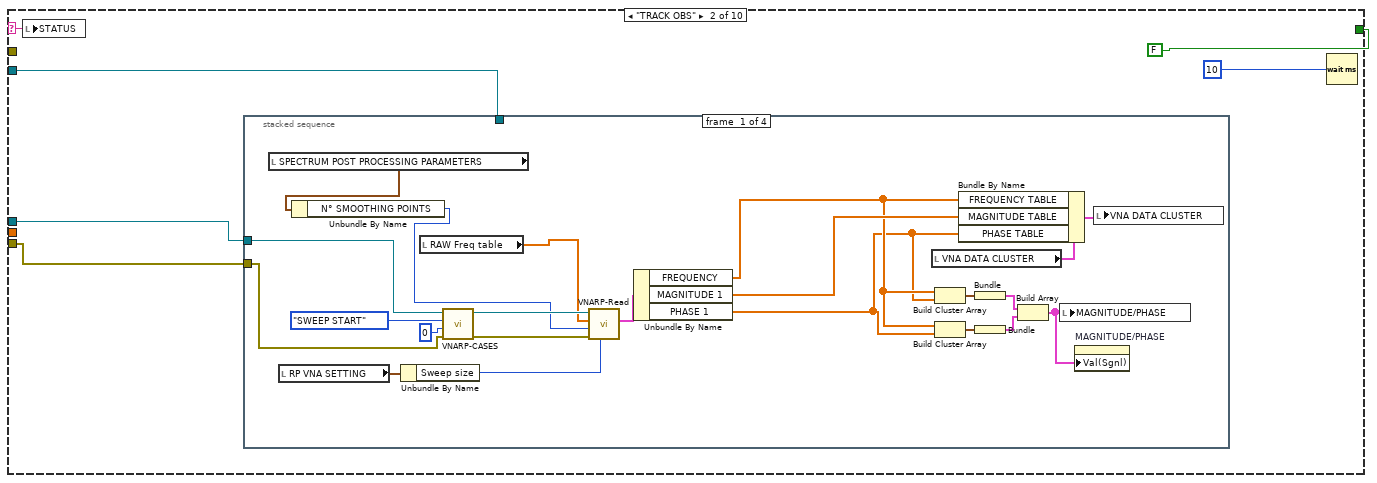
[diagram p13: hidden frame]
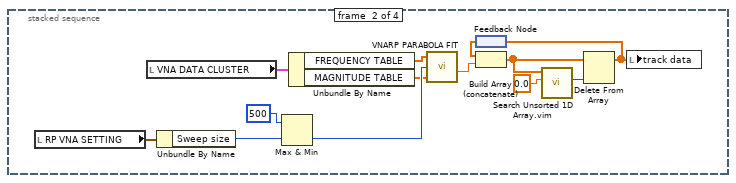
[diagram p14: hidden frame]
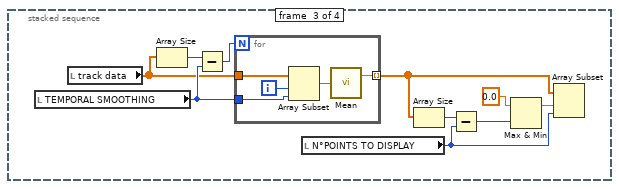
[diagram p15: hidden frame]
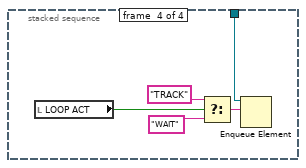
[diagram p16: hidden frame]
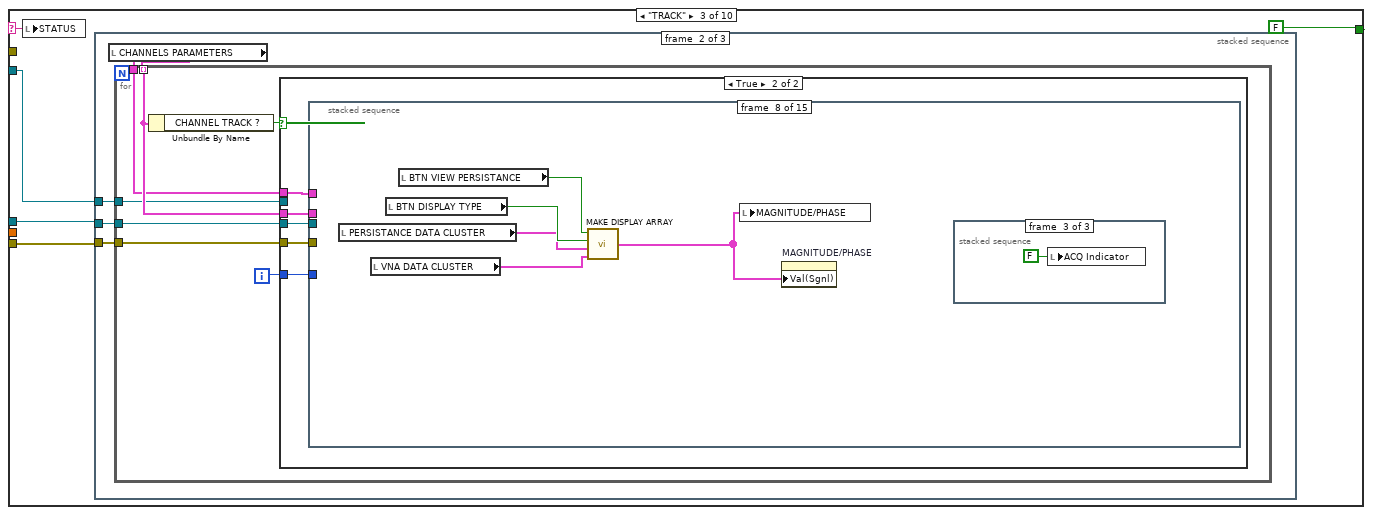
[diagram p17: hidden frame]
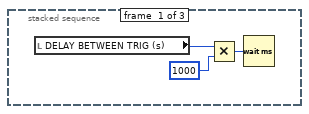
[diagram p18: hidden frame]
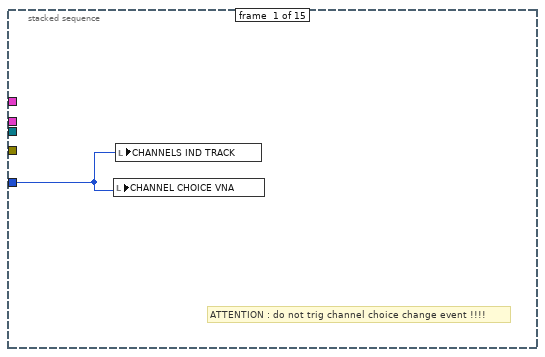
[diagram p20: hidden frame]
diagram:
  n1 = stacked-sequence {
    frame #0 {
    }
    frame #1 {
      w23 = TRUE ("x")
      w24 = 100.0 ("PUMP")
      w27 = 1900.0 ("Center")
      w28 = 1050.0 ("Center")
      w43 = u32 1000 ("Decimation")
      w41 = u32 2000000 ("Decimation")
      w42 = u32 200000 ("Decimation")
      # "INIT"
      n2 = local write "RP CONNECT"(FALSE) -> ()
      n3 = Not(x=w23) -> ()  [unwired: 1 out]
      n4 = local write "Hide/Show track data channel"(bool[] [TRUE, TRUE, TRUE, TRUE, TRUE, TRUE, TRUE, TRUE, TRUE, TRUE, TRUE, TRUE, TRUE, TRUE, TRUE, TRUE] ("Hide/Show track data channel")) -> ()
      n5 = property on="BTN PAUSE TRACK" class="Bool (strict)"("Visible"=w23) -> ()  [unwired: 2 in, 2 out]
      n6 = property on="BTN RUN TRACK" class="Bool (strict)"("Visible"=w23) -> ()  [unwired: 2 in, 2 out]
      n7 = local read "RP VNA SETTING"() -> (w45:T1)
      n8 = local read "Points N°"() -> (w26:i32)
      n9 = property on="MAIN TAB" class="TabCtl (strict)"("Tabs Visible?"=FALSE ("Onglets visibles ?")) -> ()  [unwired: 2 in, 2 out]
      n10 = local write "SPAN"(w27) -> ()
      n11 = local write "RAW Freq table"(dbl[] [200000.0, 201801.8018018018, 203603.6036036036, 205405.4054054054, 207207.20720720722, 209009.009009009, 210810.8108108108, 212612.6126126126, 214414.4144144144, 216216.2162162162, 218018.01801801802, 219819.81981981982, 221621.62162162163, 223423.42342342343, 225225.22522522524, 227027.02702702704, 228828.82882882882, 230630.63063063062, 232432.43243243243, 234234.23423423423, 236036.03603603604, 237837.83783783784, 239639.63963963964, 241441.44144144145, 243243.24324324325, 245045.04504504503, 246846.84684684683, 248648.64864864864, 250450.45045045044, 252252.25225225225, 254054.05405405405, 255855.85585585586, 257657.65765765766, 259459.45945945947, 261261.26126126124, 263063.0630630631, 264864.86486486485, 266666.6666666666, 268468.46846846846, 270270.2702702703, 272072.0720720721, 273873.87387387385, 275675.6756756757, 277477.47747747746, 279279.2792792793, 281081.08108108107, 282882.8828828829, 284684.6846846847, 286486.4864864865, 288288.2882882883, 290090.09009009006, 291891.8918918919, 293693.69369369367, 295495.4954954955, 297297.2972972973, 299099.0990990991, 300900.9009009009, 302702.7027027027, 304504.5045045045, 306306.3063063063, 308108.1081081081, 309909.90990990994, 311711.7117117117, 313513.5135135135, 315315.3153153153, 317117.1171171171, 318918.91891891893, 320720.7207207207, 322522.5225225225, 324324.3243243243, 326126.12612612615, 327927.9279279279, 329729.7297297297, 331531.53153153154, 333333.3333333333, 335135.13513513515, 336936.9369369369, 338738.7387387387, 340540.54054054053, 342342.34234234237, 344144.14414414414, 345945.9459459459, 347747.74774774775, 349549.5495495496, 351351.35135135136, 353153.15315315314, 354954.9549549549, 356756.75675675675, 358558.5585585586, 360360.36036036036, 362162.16216216213, 363963.96396396396, 365765.7657657658, 367567.5675675676, 369369.36936936935, 371171.1711711711, 372972.97297297296, 374774.7747747748, 376576.57657657657, 378378.37837837834, 380180.1801801802, 381981.981981982, 383783.7837837838, 385585.58558558556, 387387.38738738734, 389189.1891891892, 390990.990990991, 392792.7927927928, 394594.59459459456, 396396.3963963964, 398198.1981981982, 400000.0, 401801.8018018018, 403603.6036036036, 405405.4054054054, 407207.2072072072, 409009.009009009, 410810.81081081077, 412612.6126126126, 414414.41441441444, 416216.2162162162, 418018.018018018, 419819.8198198198, 421621.62162162166, 423423.42342342343, 425225.2252252252, 427027.027027027, 428828.8288288288, 430630.63063063065, 432432.4324324324, 434234.2342342342, 436036.03603603604, 437837.83783783787, 439639.63963963964, 441441.4414414414, 443243.2432432432, 445045.04504504503, 446846.84684684686, 448648.64864864864, 450450.4504504504, 452252.25225225225, 454054.0540540541, 455855.85585585586, 457657.65765765763, 459459.4594594594, 461261.26126126124, 463063.0630630631, 464864.86486486485, 466666.6666666666, 468468.46846846846, 470270.27027027024, 472072.0720720721, 473873.87387387385, 475675.6756756757, 477477.47747747746, 479279.2792792793, 481081.08108108107, 482882.8828828829, 484684.6846846847, 486486.48648648645, 488288.2882882883, 490090.09009009006, 491891.8918918919, 493693.69369369367, 495495.4954954955, 497297.2972972973, 499099.0990990991, 500900.9009009009, 502702.70270270266, 504504.5045045045, 506306.3063063063, 508108.1081081081, 509909.9099099099, 511711.7117117117, 513513.5135135135, 515315.3153153153, 517117.1171171171, 518918.91891891893, 520720.7207207207, 522522.5225225225, 524324.3243243243, 526126.1261261262, 527927.9279279279, 529729.7297297297, 531531.5315315316, 533333.3333333333, 535135.1351351351, 536936.9369369369, 538738.7387387387, 540540.5405405406, 542342.3423423423, 544144.1441441441, 545945.9459459459, 547747.7477477477, 549549.5495495496, 551351.3513513514, 553153.1531531531, 554954.9549549549, 556756.7567567567, 558558.5585585586, 560360.3603603604, 562162.1621621621, 563963.963963964, 565765.7657657657, 567567.5675675676, 569369.3693693693, 571171.1711711711, 572972.972972973, 574774.7747747747, 576576.5765765766, 578378.3783783783, 580180.1801801801, 581981.981981982, 583783.7837837838, 585585.5855855856, 587387.3873873875, 589189.1891891891, 590990.990990991, 592792.7927927928, 594594.5945945946, 596396.3963963964, 598198.1981981981, 600000.0, 601801.8018018018, 603603.6036036036, 605405.4054054054, 607207.2072072072, 609009.009009009, 610810.8108108108, 612612.6126126125, 614414.4144144144, 616216.2162162162, 618018.018018018, 619819.8198198199, 621621.6216216215, 623423.4234234234, 625225.2252252252, 627027.027027027, 628828.8288288289, 630630.6306306305, 632432.4324324324, 634234.2342342342, 636036.036036036, 637837.8378378379, 639639.6396396396, 641441.4414414414, 643243.2432432433, 645045.045045045, 646846.8468468469, 648648.6486486486, 650450.4504504504, 652252.2522522523, 654054.054054054, 655855.8558558559, 657657.6576576576, 659459.4594594594, 661261.2612612613, 663063.063063063, 664864.8648648649, 666666.6666666666, 668468.4684684684, 670270.2702702703, 672072.0720720721, 673873.8738738738, 675675.6756756757, 677477.4774774774, 679279.2792792793, 681081.0810810811, 682882.8828828828, 684684.6846846847, 686486.4864864864, 688288.2882882883, 690090.0900900901, 691891.8918918918, 693693.6936936937, 695495.4954954955, 697297.2972972973, 699099.099099099, 700900.9009009008, 702702.7027027027, 704504.5045045045, 706306.3063063063, 708108.1081081082, 709909.9099099098, 711711.7117117117, 713513.5135135135, 715315.3153153153, 717117.1171171172, 718918.9189189188, 720720.7207207207, 722522.5225225225, 724324.3243243243, 726126.1261261262, 727927.9279279279, 729729.7297297297, 731531.5315315315, 733333.3333333333, 735135.1351351351, 736936.9369369369, 738738.7387387387, 740540.5405405405, 742342.3423423424, 744144.1441441441, 745945.9459459459, 747747.7477477477, 749549.5495495496, 751351.3513513514, 753153.1531531531, 754954.9549549549, 756756.7567567567, 758558.5585585586, 760360.3603603604, 762162.1621621621, 763963.9639639639, 765765.7657657658, 767567.5675675676, 769369.3693693693, 771171.1711711711, 772972.9729729729, 774774.7747747748, 776576.5765765766, 778378.3783783783, 780180.1801801801, 781981.981981982, 783783.7837837838, 785585.5855855856, 787387.3873873873, 789189.1891891891, 790990.990990991, 792792.7927927928, 794594.5945945946, 796396.3963963963, 798198.1981981982, 800000.0, 801801.8018018018, 803603.6036036036, 805405.4054054053, 807207.2072072072, 809009.009009009, 810810.8108108108, 812612.6126126125, 814414.4144144144, 816216.2162162162, 818018.018018018, 819819.8198198198, 821621.6216216215, 823423.4234234234, 825225.2252252252, 827027.027027027, 828828.8288288288, 830630.6306306307, 832432.4324324324, 834234.2342342342, 836036.036036036, 837837.8378378379, 839639.6396396396, 841441.4414414414, 843243.2432432432, 845045.045045045, 846846.8468468469, 848648.6486486486, 850450.4504504504, 852252.2522522522, 854054.0540540541, 855855.8558558559, 857657.6576576576, 859459.4594594594, 861261.2612612612, 863063.0630630631, 864864.8648648649, 866666.6666666666, 868468.4684684684, 870270.2702702703, 872072.0720720721, 873873.8738738738, 875675.6756756756, 877477.4774774774, 879279.2792792793, 881081.0810810811, 882882.8828828828, 884684.6846846846, 886486.4864864865, 888288.2882882883, 890090.0900900901, 891891.8918918918, 893693.6936936936, 895495.4954954955, 897297.2972972973, 899099.099099099, 900900.9009009008, 902702.7027027027, 904504.5045045045, 906306.3063063063, 908108.108108108, 909909.9099099098, 911711.7117117117, 913513.5135135135, 915315.3153153153, 917117.117117117, 918918.9189189189, 920720.7207207207, 922522.5225225225, 924324.3243243243, 926126.1261261262, 927927.9279279279, 929729.7297297297, 931531.5315315315, 933333.3333333333, 935135.1351351351, 936936.9369369369, 938738.7387387387, 940540.5405405405, 942342.3423423424, 944144.1441441441, 945945.9459459459, 947747.7477477477, 949549.5495495495, 951351.3513513514, 953153.1531531531, 954954.9549549549, 956756.7567567567, 958558.5585585586, 960360.3603603604, 962162.1621621621, 963963.9639639639, 965765.7657657657, 967567.5675675676, 969369.3693693693, 971171.1711711711, 972972.9729729729, 974774.7747747748, 976576.5765765766, 978378.3783783783, 980180.1801801801, 981981.9819819819, 983783.7837837838, 985585.5855855856, 987387.3873873873, 989189.1891891891, 990990.990990991, 992792.7927927928, 994594.5945945946, 996396.3963963963, 998198.1981981982, 1000000.0, 1001801.8018018018, 1003603.6036036036, 1005405.4054054053, 1007207.2072072072, 1009009.009009009, 1010810.8108108108, 1012612.6126126125, 1014414.4144144144, 1016216.2162162162, 1018018.018018018, 1019819.8198198198, 1021621.6216216215, 1023423.4234234234, 1025225.2252252252, 1027027.027027027, 1028828.8288288288, 1030630.6306306307, 1032432.4324324324, 1034234.2342342342, 1036036.036036036, 1037837.8378378378, 1039639.6396396396, 1041441.4414414414, 1043243.2432432432, 1045045.045045045, 1046846.8468468469, 1048648.6486486485, 1050450.4504504504, 1052252.2522522523, 1054054.054054054, 1055855.8558558559, 1057657.6576576577, 1059459.4594594594, 1061261.261261261, 1063063.0630630632, 1064864.8648648649, 1066666.6666666665, 1068468.4684684684, 1070270.2702702703, 1072072.072072072, 1073873.8738738738, 1075675.6756756757, 1077477.4774774774, 1079279.2792792793, 1081081.0810810812, 1082882.8828828828, 1084684.6846846845, 1086486.4864864866, 1088288.2882882883, 1090090.09009009, 1091891.8918918918, 1093693.6936936937, 1095495.4954954954, 1097297.2972972973, 1099099.0990990992, 1100900.9009009008, 1102702.7027027027, 1104504.5045045046, 1106306.3063063063, 1108108.108108108, 1109909.9099099098, 1111711.7117117117, 1113513.5135135134, 1115315.3153153153, 1117117.1171171172, 1118918.9189189188, 1120720.7207207207, 1122522.5225225226, 1124324.3243243243, 1126126.126126126, 1127927.927927928, 1129729.7297297297, 1131531.5315315314, 1133333.3333333333, 1135135.1351351351, 1136936.9369369368, 1138738.7387387387, 1140540.5405405406, 1142342.3423423423, 1144144.1441441441, 1145945.945945946, 1147747.7477477477, 1149549.5495495494, 1151351.3513513515, 1153153.1531531531, 1154954.9549549548, 1156756.7567567567, 1158558.5585585586, 1160360.3603603602, 1162162.1621621621, 1163963.963963964, 1165765.7657657657, 1167567.5675675676, 1169369.3693693695, 1171171.1711711711, 1172972.9729729728, 1174774.774774775, 1176576.5765765766, 1178378.3783783782, 1180180.1801801801, 1181981.981981982, 1183783.7837837837, 1185585.5855855856, 1187387.3873873875, 1189189.189189189, 1190990.990990991, 1192792.792792793, 1194594.5945945946, 1196396.3963963962, 1198198.198198198, 1200000.0, 1201801.8018018017, 1203603.6036036036, 1205405.4054054054, 1207207.207207207, 1209009.009009009, 1210810.810810811, 1212612.6126126125, 1214414.4144144142, 1216216.2162162163, 1218018.018018018, 1219819.8198198196, 1221621.6216216215, 1223423.4234234234, 1225225.225225225, 1227027.027027027, 1228828.8288288289, 1230630.6306306305, 1232432.4324324324, 1234234.2342342343, 1236036.036036036, 1237837.8378378376, 1239639.6396396398, 1241441.4414414414, 1243243.243243243, 1245045.045045045, 1246846.8468468469, 1248648.6486486485, 1250450.4504504504, 1252252.2522522523, 1254054.054054054, 1255855.8558558559, 1257657.6576576575, 1259459.4594594594, 1261261.2612612613, 1263063.063063063, 1264864.8648648649, 1266666.6666666665, 1268468.4684684684, 1270270.2702702703, 1272072.072072072, 1273873.8738738738, 1275675.6756756757, 1277477.4774774774, 1279279.2792792793, 1281081.081081081, 1282882.8828828828, 1284684.6846846847, 1286486.4864864864, 1288288.2882882883, 1290090.09009009, 1291891.8918918918, 1293693.6936936937, 1295495.4954954954, 1297297.2972972973, 1299099.0990990992, 1300900.9009009008, 1302702.7027027027, 1304504.5045045044, 1306306.3063063063, 1308108.1081081082, 1309909.9099099098, 1311711.7117117117, 1313513.5135135134, 1315315.3153153153, 1317117.1171171172, 1318918.9189189188, 1320720.7207207207, 1322522.5225225224, 1324324.3243243243, 1326126.1261261262, 1327927.9279279278, 1329729.7297297297, 1331531.5315315316, 1333333.3333333333, 1335135.1351351351, 1336936.9369369368, 1338738.7387387387, 1340540.5405405406, 1342342.3423423423, 1344144.1441441441, 1345945.9459459458, 1347747.7477477477, 1349549.5495495496, 1351351.3513513512, 1353153.1531531531, 1354954.9549549548, 1356756.7567567567, 1358558.5585585586, 1360360.3603603602, 1362162.1621621621, 1363963.963963964, 1365765.7657657657, 1367567.5675675676, 1369369.3693693692, 1371171.1711711711, 1372972.972972973, 1374774.7747747747, 1376576.5765765766, 1378378.3783783782, 1380180.1801801801, 1381981.981981982, 1383783.7837837837, 1385585.5855855856, 1387387.3873873875, 1389189.189189189, 1390990.990990991, 1392792.7927927927, 1394594.5945945946, 1396396.3963963964, 1398198.198198198, 1400000.0, 1401801.8018018017, 1403603.6036036036, 1405405.4054054054, 1407207.207207207, 1409009.009009009, 1410810.8108108107, 1412612.6126126125, 1414414.4144144144, 1416216.216216216, 1418018.018018018, 1419819.8198198199, 1421621.6216216215, 1423423.4234234234, 1425225.225225225, 1427027.027027027, 1428828.8288288289, 1430630.6306306305, 1432432.4324324324, 1434234.234234234, 1436036.036036036, 1437837.8378378379, 1439639.6396396395, 1441441.4414414414, 1443243.243243243, 1445045.045045045, 1446846.8468468469, 1448648.6486486485, 1450450.4504504504, 1452252.2522522523, 1454054.054054054, 1455855.8558558559, 1457657.6576576575, 1459459.4594594594, 1461261.2612612613, 1463063.063063063, 1464864.8648648649, 1466666.6666666665, 1468468.4684684684, 1470270.2702702703, 1472072.072072072, 1473873.8738738738, 1475675.6756756757, 1477477.4774774774, 1479279.2792792793, 1481081.081081081, 1482882.8828828828, 1484684.6846846847, 1486486.4864864864, 1488288.2882882883, 1490090.09009009, 1491891.8918918918, 1493693.6936936937, 1495495.4954954954, 1497297.2972972973, 1499099.099099099, 1500900.9009009008, 1502702.7027027027, 1504504.5045045044, 1506306.3063063063, 1508108.1081081082, 1509909.9099099098, 1511711.7117117117, 1513513.5135135134, 1515315.3153153153, 1517117.1171171172, 1518918.9189189188, 1520720.7207207207, 1522522.5225225224, 1524324.3243243243, 1526126.1261261262, 1527927.9279279278, 1529729.7297297297, 1531531.5315315314, 1533333.3333333333, 1535135.1351351351, 1536936.9369369368, 1538738.7387387387, 1540540.5405405406, 1542342.3423423423, 1544144.1441441441, 1545945.9459459458, 1547747.7477477477, 1549549.5495495496, 1551351.3513513512, 1553153.1531531531, 1554954.9549549548, 1556756.7567567567, 1558558.5585585586, 1560360.3603603602, 1562162.1621621621, 1563963.963963964, 1565765.7657657657, 1567567.5675675676, 1569369.3693693692, 1571171.1711711711, 1572972.972972973, 1574774.7747747747, 1576576.5765765766, 1578378.3783783782, 1580180.1801801801, 1581981.981981982, 1583783.7837837837, 1585585.5855855856, 1587387.3873873872, 1589189.189189189, 1590990.990990991, 1592792.7927927927, 1594594.5945945946, 1596396.3963963964, 1598198.198198198, 1600000.0, 1601801.8018018017, 1603603.6036036036, 1605405.4054054054, 1607207.207207207, 1609009.009009009, 1610810.8108108107, 1612612.6126126125, 1614414.4144144144, 1616216.216216216, 1618018.018018018, 1619819.8198198196, 1621621.6216216215, 1623423.4234234234, 1625225.225225225, 1627027.027027027, 1628828.8288288289, 1630630.6306306305, 1632432.4324324324, 1634234.234234234, 1636036.036036036, 1637837.8378378379, 1639639.6396396395, 1641441.4414414414, 1643243.243243243, 1645045.045045045, 1646846.8468468469, 1648648.6486486485, 1650450.4504504504, 1652252.2522522523, 1654054.054054054, 1655855.8558558559, 1657657.6576576575, 1659459.4594594594, 1661261.2612612613, 1663063.063063063, 1664864.8648648649, 1666666.6666666665, 1668468.4684684684, 1670270.2702702703, 1672072.072072072, 1673873.8738738738, 1675675.6756756755, 1677477.4774774774, 1679279.2792792793, 1681081.081081081, 1682882.8828828828, 1684684.6846846847, 1686486.4864864864, 1688288.2882882883, 1690090.09009009, 1691891.8918918918, 1693693.6936936937, 1695495.4954954954, 1697297.2972972973, 1699099.099099099, 1700900.9009009008, 1702702.7027027027, 1704504.5045045044, 1706306.3063063063, 1708108.108108108, 1709909.9099099098, 1711711.7117117117, 1713513.5135135134, 1715315.3153153153, 1717117.1171171172, 1718918.9189189188, 1720720.7207207207, 1722522.5225225224, 1724324.3243243243, 1726126.1261261262, 1727927.9279279278, 1729729.7297297297, 1731531.5315315314, 1733333.3333333333, 1735135.1351351351, 1736936.9369369368, 1738738.7387387387, 1740540.5405405406, 1742342.3423423423, 1744144.1441441441, 1745945.9459459458, 1747747.7477477477, 1749549.5495495496, 1751351.3513513512, 1753153.1531531531, 1754954.9549549548, 1756756.7567567567, 1758558.5585585586, 1760360.3603603602, 1762162.1621621621, 1763963.9639639638, 1765765.7657657657, 1767567.5675675676, 1769369.3693693692, 1771171.1711711711, 1772972.972972973, 1774774.7747747747, 1776576.5765765766, 1778378.3783783782, 1780180.1801801801, 1781981.981981982, 1783783.7837837837, 1785585.5855855856, 1787387.3873873872, 1789189.189189189, 1790990.990990991, 1792792.7927927927, 1794594.5945945946, 1796396.3963963964, 1798198.198198198, 1800000.0, 1801801.8018018017, 1803603.6036036036, 1805405.4054054054, 1807207.207207207, 1809009.009009009, 1810810.8108108107, 1812612.6126126125, 1814414.4144144144, 1816216.216216216, 1818018.018018018, 1819819.8198198196, 1821621.6216216215, 1823423.4234234234, 1825225.225225225, 1827027.027027027, 1828828.8288288289, 1830630.6306306305, 1832432.4324324324, 1834234.234234234, 1836036.036036036, 1837837.8378378379, 1839639.6396396395, 1841441.4414414414, 1843243.243243243, 1845045.045045045, 1846846.8468468469, 1848648.6486486485, 1850450.4504504504, 1852252.252252252, 1854054.054054054, 1855855.8558558559, 1857657.6576576575, 1859459.4594594594, 1861261.2612612613, 1863063.063063063, 1864864.8648648649, 1866666.6666666665, 1868468.4684684684, 1870270.2702702703, 1872072.072072072, 1873873.8738738738, 1875675.6756756755, 1877477.4774774774, 1879279.2792792793, 1881081.081081081, 1882882.8828828828, 1884684.6846846847, 1886486.4864864864, 1888288.2882882883, 1890090.09009009, 1891891.8918918918, 1893693.6936936937, 1895495.4954954954, 1897297.2972972973, 1899099.099099099, 1900900.9009009008, 1902702.7027027027, 1904504.5045045044, 1906306.3063063063, 1908108.108108108, 1909909.9099099098, 1911711.7117117117, 1913513.5135135134, 1915315.3153153153, 1917117.1171171172, 1918918.9189189188, 1920720.7207207207, 1922522.5225225224, 1924324.3243243243, 1926126.1261261262, 1927927.9279279278, 1929729.7297297297, 1931531.5315315314, 1933333.3333333333, 1935135.1351351351, 1936936.9369369368, 1938738.7387387387, 1940540.5405405404, 1942342.3423423423, 1944144.1441441441, 1945945.9459459458, 1947747.7477477477, 1949549.5495495496, 1951351.3513513512, 1953153.1531531531, 1954954.9549549548, 1956756.7567567567, 1958558.5585585586, 1960360.3603603602, 1962162.1621621621, 1963963.9639639638, 1965765.7657657657, 1967567.5675675676, 1969369.3693693692, 1971171.1711711711, 1972972.972972973, 1974774.7747747747, 1976576.5765765766, 1978378.3783783782, 1980180.1801801801, 1981981.981981982, 1983783.7837837837, 1985585.5855855856, 1987387.3873873872, 1989189.189189189, 1990990.990990991, 1992792.7927927927, 1994594.5945945946, 1996396.3963963962, 1998198.198198198, 2000000.0] ("RAW Freq table")) -> ()
      n12 = local read "VNA SETTING CLUSTER"() -> (w32:T4)
      n13 = Divide(x=w27, y=w26) -> (x/y=w25:dbl)
      n14 = Divide(x=w42, y=w43) -> (x/y=w29:dbl)
      n15 = Divide(x=w41, y=w43) -> (x/y=w30:dbl)
      n16 = Bundle By Name(cluster=w45, "F start"=w42, "F stop"=w41, "Sweep size"=w26, "Decimation"=u32 1000, "F_corr"=u32 0, "Ph_OUT1"=u32 0, "Ph_OUT2"=u32 0 ("F_corr"), "OUT_Lvl1"=u32 32700 ("F_corr"), "OUT_Lvl2"=u32 0 ("F_corr"), "GPIO"=u32 0 ("F_corr")) -> (w44:T1)
      n17 = local write "START"(w29) -> ()
      n18 = local write "STOP"(w30) -> ()
      n19 = local write "RP VNA SETTING"(w44) -> ()
      n20 = local write "CENTER"(w28) -> ()
      n21 = Bundle By Name(cluster=w32, "START 2"=w29, "STOP 2"=w30, "CENTER 2"=w28, "SPAN 2"=w27, "PUMP"=w24, "PROBE"=w24, "Points N° 2"=w26, "SPACING 2"=w25) -> (w31:T4)
      n22 = local write "VNA SETTING CLUSTER"(w31) -> ()
      n23 = invoke on="VNA DATA CLUSTER TBL" class="Arr (strict)" method="Reinit To Default"() -> ()  [unwired: 3 in, 3 out]
      n24 = local write "CHANNELS PARAMETERS"(T10 [{"START 2"=200.0, "STOP 2"=2000.5, "CENTER 2"=1050.0, "SPAN 2"=1800.0, "CHANNEL TRACK ?"=FALSE, "PUMP"=100.0, "PROBE"=100.0, "Points N° 2"=1000, "SPACING 2"=100.0}, {"START 2"=200.0, "STOP 2"=2000.0, "CENTER 2"=1100.0, "SPAN 2"=1800.0, "CHANNEL TRACK ?"=FALSE, "PUMP"=100.0, "PROBE"=100.0, "Points N° 2"=1000, "SPACING 2"=1800.0}, {"START 2"=200.0, "STOP 2"=2000.0, "CENTER 2"=1100.0, "SPAN 2"=1800.0, "CHANNEL TRACK ?"=FALSE, "PUMP"=100.0, "PROBE"=100.0, "Points N° 2"=1000, "SPACING 2"=1800.0}, {"START 2"=200.0, "STOP 2"=2000.0, "CENTER 2"=1100.0, "SPAN 2"=1800.0, "CHANNEL TRACK ?"=FALSE, "PUMP"=100.0, "PROBE"=100.0, "Points N° 2"=1000, "SPACING 2"=1800.0}, {"START 2"=200.0, "STOP 2"=2000.0, "CENTER 2"=1100.0, "SPAN 2"=1800.0, "CHANNEL TRACK ?"=FALSE, "PUMP"=100.0, "PROBE"=100.0, "Points N° 2"=1000, "SPACING 2"=1800.0}, {"START 2"=200.0, "STOP 2"=2000.0, "CENTER 2"=1100.0, "SPAN 2"=1800.0, "CHANNEL TRACK ?"=FALSE, "PUMP"=100.0, "PROBE"=100.0, "Points N° 2"=1000, "SPACING 2"=1800.0}, {"START 2"=200.0, "STOP 2"=2000.0, "CENTER 2"=1100.0, "SPAN 2"=1800.0, "CHANNEL TRACK ?"=FALSE, "PUMP"=100.0, "PROBE"=100.0, "Points N° 2"=1000, "SPACING 2"=1800.0}, {"START 2"=200.0, "STOP 2"=2000.0, "CENTER 2"=1100.0, "SPAN 2"=1800.0, "CHANNEL TRACK ?"=FALSE, "PUMP"=100.0, "PROBE"=100.0, "Points N° 2"=1000, "SPACING 2"=1800.0}, {"START 2"=200.0, "STOP 2"=2000.0, "CENTER 2"=1100.0, "SPAN 2"=1800.0, "CHANNEL TRACK ?"=FALSE, "PUMP"=100.0, "PROBE"=100.0, "Points N° 2"=1000, "SPACING 2"=1800.0}, {"START 2"=200.0, "STOP 2"=2000.0, "CENTER 2"=1100.0, "SPAN 2"=1800.0, "CHANNEL TRACK ?"=FALSE, "PUMP"=100.0, "PROBE"=100.0, "Points N° 2"=1000, "SPACING 2"=1800.0}, {"START 2"=200.0, "STOP 2"=2000.0, "CENTER 2"=1100.0, "SPAN 2"=1800.0, "CHANNEL TRACK ?"=FALSE, "PUMP"=100.0, "PROBE"=100.0, "Points N° 2"=1000, "SPACING 2"=1800.0}, {"START 2"=200.0, "STOP 2"=2000.0, "CENTER 2"=1100.0, "SPAN 2"=1800.0, "CHANNEL TRACK ?"=FALSE, "PUMP"=100.0, "PROBE"=100.0, "Points N° 2"=1000, "SPACING 2"=1800.0}, {"START 2"=200.0, "STOP 2"=2000.0, "CENTER 2"=1100.0, "SPAN 2"=1800.0, "CHANNEL TRACK ?"=FALSE, "PUMP"=100.0, "PROBE"=100.0, "Points N° 2"=1000, "SPACING 2"=1800.0}, {"START 2"=200.0, "STOP 2"=2000.0, "CENTER 2"=1100.0, "SPAN 2"=1800.0, "CHANNEL TRACK ?"=FALSE, "PUMP"=100.0, "PROBE"=100.0, "Points N° 2"=1000, "SPACING 2"=1800.0}, {"START 2"=200.0, "STOP 2"=2000.0, "CENTER 2"=1100.0, "SPAN 2"=1800.0, "CHANNEL TRACK ?"=FALSE, "PUMP"=100.0, "PROBE"=100.0, "Points N° 2"=1000, "SPACING 2"=1800.0}, {"START 2"=200.0, "STOP 2"=2000.0, "CENTER 2"=1100.0, "SPAN 2"=1800.0, "CHANNEL TRACK ?"=FALSE, "PUMP"=100.0, "PROBE"=100.0, "Points N° 2"=1000, "SPACING 2"=1800.0}] ("CHANNELS PARAMETERS")) -> ()
      n25 = local read "TRACK DATA PARAMETERS"() -> (w19:cluster{"MAIN FOLDER":path})
      n26 = local read "TRACK DATA PARAMETERS"() -> (w4:cluster{"MAIN FOLDER":path})
      n27 = Unbundle By Name(w19) -> ("MAIN FOLDER"=w18:path)
      n28 = Unbundle By Name(w4) -> ("MAIN FOLDER"=w5:path)
      n29 = Build Path(base path=w18, name or relative path=path "Configuration file/conf.ini") -> (appended path=w16:path)
      n30 = Build Path(base path=w5, name or relative path=path "VOA calibration/PUMP.txt") -> (appended path=w8:path)
      n31 = Build Path(base path=w5, name or relative path=path "VOA calibration/PROBE.txt") -> (appended path=w9:path)
      n32 = local read "NETWORK PARAMETERS"() -> (w15:T8)
      n33 = call "RP - READ MAC CONF FILE.vi"("Path"=w16) -> ("RP2 MAC"=w13:string, "RP1 MAC"=w14:string)  [unwired: 8 in, 1 out]
      n34 = call "RP-VOA CALIBRATION FIT.vi"("file path"=w8) -> ("Calibration array"=w10:dbl[])  [unwired: 2 in, 1 out]
      n35 = call "RP-VOA CALIBRATION FIT.vi"("file path"=w9) -> ("Calibration array"=w11:dbl[])  [unwired: 2 in, 1 out]
      n36 = local read "VOA Calibration cluster"() -> (w6:cluster{"PUMP":dbl[], "PROBE":dbl[]})
      n37 = Bundle By Name(cluster=w15, "RP-MAC 1"=w14, "RP-MAC 2"=w13) -> (w12:T8)
      n38 = Bundle By Name(cluster=w6, "PUMP"=w10, "PROBE"=w11) -> (w7:cluster{"PUMP":dbl[], "PROBE":dbl[]})
      n39 = local write "NETWORK PARAMETERS"(w12) -> ()
      n40 = local write "VOA Calibration cluster"(w7) -> ()
    }
    frame #2 {
      # "CONNEXION WAIT"
      n41 = local read "NETWORK PARAMETERS"() -> (w51:T8)
      n42 = Unbundle By Name(w51) -> ("RP-MAC 1"=w50:string, "RP-MAC 2"=w49:string)
      n43 = call "RP-GET IP ADDRESS.vi"("MAC address"=w50) -> ("IP address"=w56:string)
      n44 = call "RP-GET IP ADDRESS.vi"("MAC address"=w49) -> ("IP address"=w53:string)
      n45 = local read "ENABLE INTERNAL MODULATION"() -> (w47:bool)
      n46 = Bundle By Name(cluster=w51, "RP-IP 1"=w56, "RP-IP 2"=w53) -> (w60:T8)
      n47 = String Length(string=w56) -> (length=w58:i32)
      n48 = String Length(string=w53) -> (length=w59:i32)
      n49 = call "VNARP - LAUNCH.vi"("RP IP"=w56) -> ("VNA launched ?"=w57:bool)  [unwired: 10 in]
      n50 = call "RP-START SCPI.vi"("RP IP"=w53) -> ("SCPI launched ?"=w52:bool)  [unwired: 10 in]
      n51 = Greater Than 0?(x=w58) -> (x > 0?=w55:bool)
      n52 = Greater Than 0?(x=w59) -> (x > 0?=w54:bool)
      n53 = local write "NETWORK PARAMETERS"(w60) -> ()
      n54 = Compound Arithmetic op=AND(w55, w54, w57, w52) -> (w46:bool)
      n55 = And(x=w46, y=w47) -> (x .and. y?=w48:bool)
      n56 = local write "RP CONNECT"(w46) -> ()
      n57 = case shown="True" w48 {
        frame False {
        }
        frame True {
          w63 = u16 1 items=["Channel 1"=1, "Channel 2"=2] ("Channel (1|2)")
          n58 = local read "NETWORK PARAMETERS"() -> (w62:T8)
          n59 = Unbundle By Name(w62) -> ("RP-IP 2"=w61:string)
          n60 = call "RP-GEN SINUS-OUT.vi"("Amplitude(1V)"="Amplitude(1V)", "Frequency (Hz)"=10000000, "Channel (1|2)"=w63, "IP address"=w61) -> ()  [unwired: 1 out]
        }
      }
    }
    frame #3 {
      w79 = ""  # données (peuvent avoir n'importe quel type)
      # "attente libération des deux piles avant fermeture"
      # "MAIN"
      n61 = local read "NETWORK PARAMETERS"() -> (w68:T8)
      n62 = local read "RP VNA SETTING"() -> (w75:T1)
      n63 = Unbundle By Name(w68) -> ("RP-IP 1"=w67:string)
      n64 = call "VNARP-Connexion.vi"("IP RP"=w67) -> ("sortie d'erreur"=w77:errorcluster, "ID de connexion"=w76:refnum<k5>)  [unwired: 1 in]
      n65 = Obtain Queue(element data type=w79) -> (queue out=w78:refnum<queue>, error out=w81:errorcluster)  [unwired: 4 in, 1 out]
      n66 = call "VNARP-SettingsUpdate.vi"("Error IN"=w77, "RP VNA SETTINGS IN"=w75, "ID de connexion IN"=w76) -> ("Error OUT"=w72:errorcluster, "Freq table"=w73:dbl[], "ID de connexion OUT"=w74:refnum<k5>)
      n67 = while {
        shift-right: [w606] -> w80
        shift-left: w81 -> [w608]
        tunnel: w78 -> [w609]
        tunnel: [w604] -> w71
        stop <- w604 stop-if-true
        n68 = event shown="[24] \"BTN VIEW PERSISTANCE\": Value Change" {
          selector: _ -> [_ _ _ _ _ _ _ _ _ _ _ _ _ _ _ _ _ _ _ _ _ _ _ _ _ _]
          dyn-events: _ -> [_ _ _ _ _ _ _ _ _ _ _ _ _ _ _ _ _ _ _ _ _ _ _ _ _ _]
          timeout: 250 -> [_ _ _ _ _ _ _ _ _ _ _ _ _ _ _ _ _ _ _ _ _ _ _ _ _ _]
          tunnel: w609 -> [w614 w617 w621 _ _ w652 _ w677 w699 w725 w751 w774 w786 w815 _ _ _ _ _ w828 _ w854 _ w862 _ _]
          tunnel: w608 -> [w612 w616 w620 _ _ w651 _ w676 w698 w724 w753 w773 w785 w814 _ _ _ _ _ w827 _ w855 _ w861 _ _]
          tunnel: [w611 w615 w619 _ _ w650 _ w675 w697 w722 w752 w772 w784 w816 _ _ _ _ _ w826 _ w853 _ w860 _ _] -> w606
          tunnel: [_ _ _ _ _ _ _ _ _ _ _ _ _ w812 _ _ _ _ _ _ _ _ _ _ _ _] -> w607
          event "BTN LOOP VNA": Value Change {
            n69 = event-data() -> ("NewVal"=w610:bool)  [unwired: 1 in]
            n70 = local write "LOOP ACT"(w610) -> ()
            n71 = Enqueue Element(queue=w614, element="VNA LOOP", error in (no error)=w612) -> (error out=w611:errorcluster)  [unwired: 1 in, 2 out]
          }
          event "BTN RUN VNA": Mouse Up {
            n72 = event-data() -> ()  [unwired: 1 in, 2 out]
            n73 = Enqueue Element(queue=w617, element="RUN VNA", error in (no error)=w616) -> (error out=w615:errorcluster)  [unwired: 1 in, 2 out]
          }
          event "PUMP", "PROBE": Mouse Up {
            n74 = event-data() -> ()  [unwired: 1 in, 2 out]
            n75 = Enqueue Element(queue=w621, element="POWER UPDATE", error in (no error)=w620) -> (error out=w619:errorcluster)  [unwired: 1 in, 2 out]
          }
          event "Hide/Show track data channel": Value Change {
            # "TO TEST ON ALPHA"
            n76 = event-data() -> ()  [unwired: 1 in, 2 out]
            n77 = local read "Hide/Show track data channel"() -> (w623:bool[])
            n78 = for {
              tunnel: w623 -> [w624] mode=indexing
              i -> [w625]
              n79 = flat-sequence {
                tunnel: w625 -> [w626]
                tunnel: w624 -> [w627]
                frame #0 {
                  n80 = property on="LIVE TRACK" class="WFGraph (strict)"("Active Plot"=w626) -> ()  [unwired: 2 in, 2 out]
                }
                frame #1 {
                  n81 = property on="LIVE TRACK" class="WFGraph (strict)"("Plot.Visible?"=w627) -> ()  [unwired: 2 in, 2 out]
                }
              }
            }
          }
          event "MAGNITUDE/PHASE": Value Change {
            n82 = event-data() -> ()  [unwired: 1 in, 2 out]
            n83 = local read "BTN AUTOSCALE"() -> (w632:bool)
            n84 = case shown="True" w632 {
              frame False {
              }
              frame True {
                n85 = flat-sequence {
                  frame #0 {
                    n86 = property on="MAGNITUDE/PHASE" class="XYGraph (strict)"("ActYScl"=0 ("Active Y Scale")) -> ()  [unwired: 2 in, 2 out]
                  }
                  frame #1 {
                    n87 = local read "BTN DISPLAY TYPE"() -> (w634:bool)
                    n88 = case shown="False" w634 {
                      frame False {
                        n89 = local read "PERSISTANCE DATA CLUSTER"() -> (w641:T9)
                        n90 = local read "VNA DATA CLUSTER"() -> (w646:T9)
                        n91 = local read "BTN VIEW PERSISTANCE"() -> (w638:bool)
                        n92 = Unbundle By Name(w641) -> ("MAGNITUDE TABLE"=w642:ext[])
                        n93 = Unbundle By Name(w646) -> ("MAGNITUDE TABLE"=w647:ext[])
                        n94 = Array Max & Min(array=w642) -> (max value=w636:ext)  [unwired: 3 out]
                        n95 = Array Max & Min(array=w647) -> (max value=w640:ext)  [unwired: 3 out]
                        n96 = Select(t=w636, s=w638, f=0.0 ("t")) -> (s? t:f=w637:ext)
                        n97 = Max & Min(x=w640, y=w637) -> (max(x,y)=w639:ext)  [unwired: 1 out]
                        n98 = Multiply(x=1.1, y=w639) -> (x*y=w644:ext)
                        n99 = property on="MAGNITUDE/PHASE" class="XYGraph (strict)"("YScale.Maximum"=w644, "YScale.Minimum"=0.0) -> ()  [unwired: 2 in, 2 out]
                      }
                      frame True {
                        n100 = property on="MAGNITUDE/PHASE" class="XYGraph (strict)"("YScale.ScaleFit"=u8 1 ("Y Scale.Scale Fit")) -> ()  [unwired: 2 in, 2 out]
                      }
                    }
                  }
                }
              }
            }
            n101 = local read "BTN DISPLAY TYPE"() -> (w629:bool)
            n102 = Select(t="I/Q", s=w629, f="MAGNITUDE/PHASE") -> (s? t:f=w628:string)
            n103 = property on="MAGNITUDE/PHASE" class="XYGraph (strict)"("Caption.Text"=w628) -> ()  [unwired: 2 in, 2 out]
          }
          event "CHANNEL CHOICE VNA": Value Change {
            n104 = event-data() -> ()  [unwired: 1 in, 2 out]
            n105 = Enqueue Element(queue=w652, element="CHANNEL CHANGE", error in (no error)=w651) -> (error out=w650:errorcluster)  [unwired: 1 in, 2 out]
            n106 = One Button Dialog(message="TRIGGERED !") -> ()  [unwired: 1 in, 1 out]
          }
          event "BTN NEW TRACK": Mouse Up {
            n107 = event-data() -> ()  [unwired: 1 in, 2 out]
            n108 = Two Button Dialog(message="Initiate a new tracking session ?") -> (T button?=w654:bool)  [unwired: 2 in]
            n109 = case shown="True" w654 {
              frame False {
              }
              frame True {
                n110 = stacked-sequence {
                  frame #0 {
                    # "LOCK ALL CONTROLS"
                  }
                  frame #1 {
                    n111 = local read "ASSAY NAME"() -> (w661:string)
                    n112 = local read "CHANNELS PARAMETERS"() -> (w662:T4[])
                    n113 = local read "TRACK DATA PARAMETERS"() -> (w660:cluster{"MAIN FOLDER":path})
                    n114 = Unbundle By Name(w660) -> ("MAIN FOLDER"=w659:path)
                    n115 = call "RP-TRACKDataStructBuild.vi"("CHANNELS PARAMETERS"=w662, "Track session name"=w661, "SensWay track data path"=w659) -> ("TRACK REPOSITERY"=w658:path, "Track File List"=w657:path[], "Track Repositery List"=w656:path[])
                    n116 = local write "Track Repositery List"(w656) -> ()
                    n117 = local write "Track File List"(w657) -> ()
                    n118 = local write "TRACK REPOSITERY"(w658) -> ()
                  }
                  frame #2 {
                    n119 = local read "CHANNELS PARAMETERS"() -> (w664:T4[])
                    n120 = for {
                      tunnel: w664 -> [w674] mode=indexing
                      border: cluster{"CHANNEL":dbl, "KPI 1 TRACK":ext[]}[] [] -> [_]
                      i -> [w670]
                      n121 = Unbundle By Name(w674) -> ("CHANNEL TRACK ?"=w665:bool)
                      n122 = Select(t=dbl[] [0.0], s=w665, f=dbl[] []) -> (s? t:f=w668:dbl[])
                      n123 = Bundle By Name(cluster=cluster{"CHANNEL":dbl, "KPI 1 TRACK":ext[]} {"CHANNEL"=0.0, "KPI 1 TRACK"=[0.0]} ("TRACK DATA CLUSTER"), "CHANNEL"=w670, "KPI 1 TRACK"=w668) -> (w669:cluster{"CHANNEL":dbl, "KPI 1 TRACK":ext[]})
                      n124 = feedback #1() -> (w672:cluster{"CHANNEL":dbl, "KPI 1 TRACK":ext[]}[])
                      n125 = Build Array (concatenate)(w672, w669) -> (w673:cluster{"CHANNEL":dbl, "KPI 1 TRACK":ext[]}[])
                      n126 = feedback-in #1(w673) -> ()
                      n127 = local write "TRACK DATA CLUSTER TBL"(w673) -> ()
                    }
                  }
                  frame #3 {
                  }
                }
              }
            }
          }
          event "START", "STOP": Value Change {
            n128 = event-data() -> ()  [unwired: 1 in, 1 out]
            n129 = stacked-sequence {
              frame #0 {
                n130 = local read "STOP"() -> (w683:dbl)
                n131 = local read "START"() -> (w682:dbl)
                n132 = Subtract(x=w683, y=w682) -> (x-y=w684:dbl)
                n133 = Add(x=w683, y=w682) -> (x+y=w681:dbl)
                n134 = local write "SPAN"(w684) -> ()
                n135 = Divide(x=w681, y=2.0) -> (x/y=w679:dbl)
                n136 = local write "CENTER"(w679) -> ()
              }
              frame #1 {
                n137 = local read "Points N°"() -> (w689:i32)
                n138 = local read "SPAN"() -> (w688:dbl)
                n139 = Divide(x=w688, y=w689) -> (x/y=w687:dbl)
                n140 = Multiply(x=w687, y=1000.0) -> (x*y=w686:dbl)
                n141 = local write "SPACING"(w686) -> ()
              }
              frame #2 {
                w690 = 1000
                n142 = local read "STOP"() -> (w692:dbl)
                n143 = local read "START"() -> (w694:dbl)
                n144 = Multiply(x=w694, y=w690) -> (x*y=w693:dbl)
                n145 = Multiply(x=w690, y=w692) -> (x*y=w691:dbl)
                n146 = local read "RP VNA SETTING"() -> (w696:T1)
                n147 = Bundle By Name(cluster=w696, "F start"=w693, "F stop"=w691) -> (w695:T1)
                n148 = local write "RP VNA SETTING"(w695) -> ()
              }
            }
            n149 = Enqueue Element(queue=w677, element="UPDATE", error in (no error)=w676) -> (error out=w675:errorcluster)  [unwired: 1 in, 2 out]
          }
          event "CENTER", "SPAN": Value Change {
            n150 = event-data() -> ()  [unwired: 1 in, 1 out]
            n151 = stacked-sequence {
              frame #0 {
                w702 = 100.0 ("y")
                n152 = local read "CENTER"() -> (w706:dbl)
                n153 = local read "SPAN"() -> (w708:dbl)
                n154 = Divide(x=w708, y=2.0) -> (x/y=w705:dbl)
                n155 = Subtract(x=w706, y=w705) -> (x-y=w703:dbl)
                n156 = Add(x=w706, y=w705) -> (x+y=w709:dbl)
                n157 = local write "STOP"(w709) -> ()
                n158 = Greater Or Equal?(x=w703, y=w702) -> (x >= y?=w704:bool)
                n159 = Select(t=w703, s=w704, f=w702) -> (s? t:f=w701:dbl)
                n160 = local write "START"(w701) -> ()
              }
              frame #1 {
                n161 = local read "Points N°"() -> (w714:i32)
                n162 = local read "SPAN"() -> (w713:dbl)
                n163 = Divide(x=w713, y=w714) -> (x/y=w712:dbl)
                n164 = Multiply(x=w712, y=1000.0) -> (x*y=w711:dbl)
                n165 = local write "SPACING"(w711) -> ()
              }
              frame #2 {
                w715 = 1000
                n166 = local read "STOP"() -> (w717:dbl)
                n167 = local read "START"() -> (w719:dbl)
                n168 = Multiply(x=w719, y=w715) -> (x*y=w718:dbl)
                n169 = Multiply(x=w715, y=w717) -> (x*y=w716:dbl)
                n170 = local read "RP VNA SETTING"() -> (w721:T1)
                n171 = Bundle By Name(cluster=w721, "F start"=w718, "F stop"=w716) -> (w720:T1)
                n172 = local write "RP VNA SETTING"(w720) -> ()
              }
            }
            n173 = Enqueue Element(queue=w699, element="UPDATE", error in (no error)=w698) -> (error out=w697:errorcluster)  [unwired: 1 in, 2 out]
          }
          event "BTN ZOOM+": Mouse Up; "BTN ZOOM+": Value Change {
            n174 = event-data() -> ()  [unwired: 1 in, 1 out]
            n175 = stacked-sequence {
              frame #0 {
                n176 = local read "SPAN"() -> (w728:dbl)
                n177 = Multiply(x=w728, y=0.8) -> (x*y=w726:dbl)
                n178 = local write "SPAN"(w726) -> ()
              }
              frame #1 {
                n179 = local read "Points N°"() -> (w733:i32)
                n180 = local read "SPAN"() -> (w732:dbl)
                n181 = Divide(x=w732, y=w733) -> (x/y=w731:dbl)
                n182 = Multiply(x=w731, y=1000.0) -> (x*y=w730:dbl)
                n183 = local write "SPACING"(w730) -> ()
              }
              frame #2 {
                w735 = 100.0 ("y")
                n184 = local read "SPAN"() -> (w738:dbl)
                n185 = local read "CENTER"() -> (w740:dbl)
                n186 = Divide(x=w738, y=2.0) -> (x/y=w739:dbl)
                n187 = Subtract(x=w740, y=w739) -> (x-y=w736:dbl)
                n188 = Add(x=w740, y=w739) -> (x+y=w742:dbl)
                n189 = local write "STOP"(w742) -> ()
                n190 = Greater Or Equal?(x=w736, y=w735) -> (x >= y?=w737:bool)
                n191 = Select(t=w736, s=w737, f=w735) -> (s? t:f=w734:dbl)
                n192 = local write "START"(w734) -> ()
              }
              frame #3 {
                w743 = 1000
                n193 = local read "STOP"() -> (w745:dbl)
                n194 = local read "START"() -> (w747:dbl)
                n195 = Multiply(x=w747, y=w743) -> (x*y=w746:dbl)
                n196 = Multiply(x=w743, y=w745) -> (x*y=w744:dbl)
                n197 = local read "RP VNA SETTING"() -> (w749:T1)
                n198 = Bundle By Name(cluster=w749, "F start"=w746, "F stop"=w744) -> (w748:T1)
                n199 = local write "RP VNA SETTING"(w748) -> ()
              }
            }
            n200 = Enqueue Element(queue=w725, element="UPDATE", error in (no error)=w724) -> (error out=w722:errorcluster)  [unwired: 1 in, 2 out]
          }
          event "BTN RESET VNA": Mouse Up {
            n201 = event-data() -> ()  [unwired: 1 in, 1 out]
            n202 = flat-sequence {
              tunnel: w751 -> [w755]
              tunnel: [w755] -> w750
              frame #0 {
                w764 = u32 1000 ("Decimation")
                w762 = u32 2000000 ("Decimation")
                w763 = u32 200000 ("Decimation")
                w757 = u32 32700 ("F_corr")
                n203 = local read "RP VNA SETTING"() -> (w767:T1)
                n204 = local read "Points N°"() -> (w765:i32)
                n205 = Bundle By Name(cluster=w767, "F start"=w763, "F stop"=w762, "Sweep size"=w765, "Decimation"=u32 5000, "F_corr"=u32 0, "Ph_OUT1"=u32 0, "Ph_OUT2"=u32 0 ("F_corr"), "OUT_Lvl1"=w757, "OUT_Lvl2"=w757, "GPIO"=u32 0 ("F_corr")) -> (w766:T1)
                n206 = local write "RP VNA SETTING"(w766) -> ()
                n207 = Divide(x=w762, y=w764) -> (x/y=w768:dbl)
                n208 = Divide(x=w763, y=w764) -> (x/y=w769:dbl)
                n209 = local write "CENTER"(1050.0 ("Center")) -> ()
                n210 = local write "SPAN"(1900.0 ("Center")) -> ()
                n211 = local write "START"(w769) -> ()
                n212 = local write "STOP"(w768) -> ()
              }
            }
            n213 = Enqueue Element(queue=w750, element="UPDATE", error in (no error)=w753) -> (error out=w752:errorcluster)  [unwired: 1 in, 2 out]
          }
          event "Points N°": Value Change {
            n214 = event-data() -> ()  [unwired: 1 in, 1 out]
            n215 = stacked-sequence {
              frame #0 {
                n216 = local read "Points N°"() -> (w780:i32)
                n217 = local read "SPAN"() -> (w779:dbl)
                n218 = Divide(x=w779, y=w780) -> (x/y=w778:dbl)
                n219 = Multiply(x=w778, y=1000.0) -> (x*y=w777:dbl)
                n220 = local write "SPACING"(w777) -> ()
              }
              frame #1 {
                n221 = local read "Points N°"() -> (w781:i32)
                n222 = local read "RP VNA SETTING"() -> (w783:T1)
                n223 = Bundle By Name(cluster=w783, "Sweep size"=w781) -> (w782:T1)
                n224 = local write "RP VNA SETTING"(w782) -> ()
              }
            }
            n225 = Enqueue Element(queue=w774, element="UPDATE", error in (no error)=w773) -> (error out=w772:errorcluster)  [unwired: 1 in, 2 out]
          }
          event "BTN ZOOM-": Mouse Up {
            n226 = event-data() -> ()  [unwired: 1 in, 1 out]
            n227 = stacked-sequence {
              frame #0 {
                n228 = local read "SPAN"() -> (w790:dbl)
                n229 = Multiply(x=w790, y=1.2) -> (x*y=w788:dbl)
                n230 = local write "SPAN"(w788) -> ()
              }
              frame #1 {
                n231 = local read "Points N°"() -> (w795:i32)
                n232 = local read "SPAN"() -> (w794:dbl)
                n233 = Divide(x=w794, y=w795) -> (x/y=w793:dbl)
                n234 = Multiply(x=w793, y=1000.0) -> (x*y=w792:dbl)
                n235 = local write "SPACING"(w792) -> ()
              }
              frame #2 {
                w798 = 100.0 ("y")
                n236 = local read "SPAN"() -> (w800:dbl)
                n237 = local read "CENTER"() -> (w803:dbl)
                n238 = Divide(x=w800, y=2.0) -> (x/y=w802:dbl)
                n239 = Subtract(x=w803, y=w802) -> (x-y=w796:dbl)
                n240 = Add(x=w803, y=w802) -> (x+y=w804:dbl)
                n241 = Greater Or Equal?(x=w796, y=w798) -> (x >= y?=w799:bool)
                n242 = Select(t=w796, s=w799, f=w798) -> (s? t:f=w797:dbl)
                n243 = local write "STOP"(w804) -> ()
                n244 = local write "START"(w797) -> ()
              }
              frame #3 {
                w805 = 1000
                n245 = local read "STOP"() -> (w807:dbl)
                n246 = local read "START"() -> (w809:dbl)
                n247 = Multiply(x=w809, y=w805) -> (x*y=w808:dbl)
                n248 = Multiply(x=w805, y=w807) -> (x*y=w806:dbl)
                n249 = local read "RP VNA SETTING"() -> (w811:T1)
                n250 = Bundle By Name(cluster=w811, "F start"=w808, "F stop"=w806) -> (w810:T1)
                n251 = local write "RP VNA SETTING"(w810) -> ()
              }
            }
            n252 = Enqueue Element(queue=w786, element="UPDATE", error in (no error)=w785) -> (error out=w784:errorcluster)  [unwired: 1 in, 2 out]
          }
          event "BTN STOP": Value Change {
            n253 = event-data() -> ()  [unwired: 1 in, 1 out]
            n254 = Two Button Dialog(message="Are you sure you want to exit ?") -> (T button?=w812:bool)  [unwired: 2 in]
            n255 = case shown="True" w812 {
              tunnel: [w817 w820] -> w816
              tunnel: w815 -> [_ w819]
              tunnel: w814 -> [w817 w818]
              frame False {
              }
              frame True {
                n256 = Enqueue Element(queue=w819, element="STOP", error in (no error)=w818) -> (error out=w820:errorcluster)  [unwired: 1 in, 2 out]
              }
            }
          }
          event "PANEL GENERAL SETTINGS": Value Change {
            n257 = event-data() -> ()  [unwired: 1 in, 2 out]
            n258 = local write "MAIN TAB"(enum32{"Page 1", "Page 4", "Page 2", "Page 3"}."Page 3" ("Tab Control")) -> ()
          }
          event Timeout {
            n259 = event-data() -> ()  [unwired: 1 in, 2 out]
          }
          event "PANEL TRACK SETTINGS": Value Change {
            n260 = event-data() -> ()  [unwired: 1 in, 2 out]
            n261 = local write "MAIN TAB"(enum32{"Page 1", "Page 4", "Page 2", "Page 3"}."Page 2" ("Tab Control")) -> ()
          }
          event "PANEL VNA": Value Change {
            n262 = event-data() -> ()  [unwired: 1 in, 2 out]
            n263 = local write "MAIN TAB"(enum32{"Page 1", "Page 4", "Page 2", "Page 3"}."Page 1" ("Tab Control")) -> ()
          }
          event "PANEL TRACKING": Value Change {
            n264 = event-data() -> ()  [unwired: 1 in, 2 out]
            n265 = local write "MAIN TAB"(enum32{"Page 1", "Page 4", "Page 2", "Page 3"}."Page 4" ("Tab Control")) -> ()
          }
          event "BTN Center to max": Mouse Up; "BTN Center to max": Value Change {
            n266 = event-data() -> ()  [unwired: 1 in, 2 out]
            n267 = stacked-sequence {
              frame #0 {
                # "ATTENTION ! CONFUSION  freq table"
                n268 = local read "VNA DATA CLUSTER"() -> (w833:T9)
                n269 = Unbundle By Name(w833) -> ("FREQUENCY TABLE"=w832:ext[], "MAGNITUDE TABLE"=w831:ext[])
                n270 = Array Max & Min(array=w831) -> (max index (indices)=w836:i32)  [unwired: 3 out]
                n271 = Index Array(array=w832, index=w836) -> (element=w835:ext)
                n272 = Divide(x=w835, y=1000.0) -> (x/y=w830:ext)
                n273 = local write "CENTER"(w830) -> ()
                n274 = property on="CENTER" class="DigNum (strict)"("Val(Sgnl)"=w830) -> ()  [unwired: 2 in, 2 out]
              }
              frame #1 {
                w839 = 1000
                n275 = local read "START"() -> (w837:dbl)
                n276 = local read "STOP"() -> (w838:dbl)
                n277 = Multiply(x=w837, y=w839) -> (x*y=w841:dbl)
                n278 = Multiply(x=w839, y=w838) -> (x*y=w840:dbl)
                n279 = local read "RP VNA SETTING"() -> (w843:T1)
                n280 = Bundle By Name(cluster=w843, "F start"=w841, "F stop"=w840) -> (w842:T1)
                n281 = local write "RP VNA SETTING"(w842) -> ()
              }
            }
            n282 = Enqueue Element(queue=w828, element="UPDATE", error in (no error)=w827) -> (error out=w826:errorcluster)  [unwired: 1 in, 2 out]
          }
          event "BTN AF VNA": Mouse Up {
            n283 = event-data() -> ()  [unwired: 1 in, 2 out]
            n284 = local read "AUTOFOCUS PARAMETERS"() -> (w845:cluster{"ITERATIONS":i32})
            n285 = Unbundle By Name(w845) -> ("ITERATIONS"=w844:i32)
            n286 = for {
              N: w844 -> [_]
              tunnel: [w848] -> w846
              n287 = flat-sequence {
                tunnel: [w849] -> w848
                frame #0 {
                  w849 = FALSE ("Valeur (Signalisation)")
                  n288 = property on="BTN Center to max" class="Bool (strict)"("Val(Sgnl)"=w849) -> ()  [unwired: 2 in, 2 out]
                }
                frame #1 {
                  n289 = property on="BTN ZOOM+" class="Bool (strict)"("Val(Sgnl)"=FALSE ("Valeur (Signalisation)")) -> ()  [unwired: 2 in, 2 out]
                }
              }
              n290 = Wait (ms)(milliseconds to wait=u32 250 ("attente (ms)")) -> ()  [unwired: 1 out]
            }
            n291 = property on="BTN Center to max" class="Bool (strict)"("Val(Sgnl)"=w846) -> ()  [unwired: 2 in, 2 out]
          }
          event "BTN RUN TRACK": Value Change {
            w851 = TRUE ("x")
            n292 = event-data() -> ()  [unwired: 1 in, 2 out]
            n293 = Not(x=w851) -> (.not. x?=w852:bool)
            n294 = local write "LOOP ACT"(w851) -> ()
            n295 = property on="BTN PAUSE TRACK" class="Bool (strict)"("Visible"=w851) -> ()  [unwired: 2 in, 2 out]
            n296 = Enqueue Element(queue=w854, element="TRACK", error in (no error)=w855) -> (error out=w853:errorcluster)  [unwired: 1 in, 2 out]
            n297 = property on="BTN RUN TRACK" class="Bool (strict)"("Visible"=w852) -> ()  [unwired: 2 in, 2 out]
          }
          event "BTN PAUSE TRACK": Mouse Up {
            w857 = FALSE ("x")
            n298 = event-data() -> ()  [unwired: 1 in, 2 out]
            n299 = Not(x=w857) -> (.not. x?=w858:bool)
            n300 = local write "LOOP ACT"(w857) -> ()
            n301 = property on="BTN PAUSE TRACK" class="Bool (strict)"("Visible"=w857) -> ()  [unwired: 2 in, 2 out]
            n302 = property on="BTN RUN TRACK" class="Bool (strict)"("Visible"=w858) -> ()  [unwired: 2 in, 2 out]
          }
          event "BTN SAVE VNA": Mouse Up {
            n303 = event-data() -> ()  [unwired: 1 in, 2 out]
            n304 = Enqueue Element(queue=w862, element="SAVE VNA", error in (no error)=w861) -> (error out=w860:errorcluster)  [unwired: 1 in, 2 out]
          }
          event "BTN VIEW PERSISTANCE": Value Change {
            n305 = event-data() -> ("NewVal"=w863:bool)  [unwired: 1 in, 1 out]
            n306 = case shown="True" w863 {
              frame False {
              }
              frame True {
                n307 = local read "VNA DATA CLUSTER"() -> (w864:T9)
                n308 = local write "PERSISTANCE DATA CLUSTER"(w864) -> ()
              }
            }
          }
          event "BTN DISPLAY TYPE": Value Change {
            n309 = event-data() -> ("NewVal"=w865:bool)  [unwired: 1 in, 1 out]
            n310 = case shown="True" w865 {
              frame False {
                n311 = property on="BTN FIT DISPLAY" class="Bool (strict)"("DisabledEnum"=T12."Enabled" ("Disabled")) -> ()  [unwired: 2 in, 2 out]
              }
              frame True {
                n312 = property on="BTN FIT DISPLAY" class="Bool (strict)"("DisabledEnum"=T12."Disabled and Grayed Out" ("Disabled"), "Value"=FALSE ("Fit display")) -> ()  [unwired: 2 in, 2 out]
              }
            }
          }
        }
        n313 = Or(x=w606, y=w607) -> (x .or. y?=w604:bool)
        n314 = Wait (ms)(milliseconds to wait=u32 50 ("attente (ms)")) -> ()  [unwired: 1 out]
      }
      n315 = while {
        tunnel: w78 -> [w90]
        tunnel: w74 -> [w88]
        tunnel: w73 -> [w87]
        tunnel: w72 -> [w86]
        tunnel: [w85] -> w70
        border: dbl[] [0.0] -> [_]
        stop <- w85 stop-if-true
        n316 = Dequeue Element(queue=w90) -> (queue out=w89:refnum<queue>, element=w91:string, error out=w92:errorcluster)  [unwired: 2 in, 1 out]
        n317 = case shown="No Error" w92 {
          selector: w92 -> [w97 _]
          tunnel: w91 -> [w99 _]
          tunnel: [w93 TRUE] -> w85
          tunnel: w89 -> [w98 _]
          tunnel: w88 -> [w96 _]
          tunnel: w87 -> [w95 _]
          tunnel: w86 -> [w94 _]
          frame No Error {
            n318 = case shown="\"RUN VNA\"" w99 {
              selector: w99 -> [w106 w157 w217 w441 _ w520 w525 w545 _ w595]
              tunnel: w98 -> [w104 w152 w213 _ _ _ _ _ _ _]
              tunnel: w97 -> [_ _ _ _ _ _ _ _ _ _]
              tunnel: w96 -> [w103 w154 w215 w439 _ _ w524 _ _ w598]
              tunnel: w95 -> [w102 _ _ _ _ _ _ _ _ _]
              tunnel: w94 -> [w101 w153 w214 w438 _ _ w523 _ _ w597]
              tunnel: [FALSE FALSE FALSE FALSE FALSE FALSE FALSE FALSE FALSE TRUE] -> w93
              frame "VNA LOOP", Default {
                n319 = local write "STATUS"(w106) -> ()
                n320 = stacked-sequence {
                  tunnel: w103 -> [w119 _ _]
                  tunnel: w102 -> [_ _ _]
                  tunnel: w101 -> [w118 _ _]
                  tunnel: w104 -> [_ _ w148]
                  frame #0 {
                    n321 = local read "SPECTRUM POST PROCESSING PARAMETERS"() -> (w115:cluster{"N° SMOOTHING POINTS":i32})
                    n322 = local read "RP VNA SETTING"() -> (w124:T1)
                    n323 = Unbundle By Name(w115) -> ("N° SMOOTHING POINTS"=w113:i32)
                    n324 = local read "RAW Freq table"() -> (w114:dbl[])
                    n325 = Unbundle By Name(w124) -> ("Sweep size"=w123:u32)
                    n326 = local read "VNA DATA CLUSTER"() -> (w117:T9)
                    n327 = call "VNARP-CASES.vi"("entrée d'erreur (pas d'erreur)"=w118, "Setting"=u32 0, "Énum"=T11."SWEEP START", "ID de connexion"=w119) -> ("sortie d'erreur"=w122:errorcluster, "ID de connexion en sortie"=w125:refnum<k5>)  [unwired: 3 in]
                    n328 = call "VNARP-Read.vi"("SIZE"=w123, "entrée d'erreur (pas d'erreur)"=w122, "smoothing points"=w113, "Freq table IN"=w114, "ID de connexion"=w125) -> ("DATA OUT"=w112:T13)  [unwired: 4 in, 2 out]
                    n329 = Unbundle By Name(w112) -> ("FREQUENCY"=w111:sgl[], "MAGNITUDE 1"=w110:dbl[], "PHASE 1"=w109:dbl[], "REAL 1"=w108:dbl[], "IMAGINARY 1"=w107:sgl[])
                    n330 = Bundle By Name(cluster=w117, "FREQUENCY TABLE"=w111, "MAGNITUDE TABLE"=w110, "PHASE TABLE"=w109, "REAL TABLE"=w108, "IMAGINARY TABLE"=w107) -> (w116:T9)
                    n331 = local write "VNA DATA CLUSTER"(w116) -> ()
                  }
                  frame #1 {
                    n332 = local read "PERSISTANCE DATA CLUSTER"() -> (w133:T9)
                    n333 = local read "VNA DATA CLUSTER"() -> (w130:T9)
                    n334 = local read "BTN VIEW PERSISTANCE"() -> (w132:bool)
                    n335 = local read "BTN DISPLAY TYPE"() -> (w134:bool)
                    n336 = local read "RP VNA SETTING"() -> (w131:T1)
                    n337 = local read "RESONNANCE DETECTION"() -> (w129:T6)
                    n338 = call "MAKE DISPLAY ARRAY.vi"("VNA DATA CLUSTER"=w130, "PERSISTANCE DATA CLUSTER"=w133, "Display type (F : MAG/PHASE)"=w134, "Persistance"=w132) -> ("Display array"=w127:T14)  [unwired: 2 in]
                    n339 = local read "BTN FIT DISPLAY"() -> (w128:bool)
                    n340 = case shown="True" w128 {
                      tunnel: w129 -> [_ w143]
                      tunnel: w130 -> [_ w140]
                      tunnel: w131 -> [_ w139]
                      tunnel: w127 -> [w135 w137]
                      tunnel: [w135 w136] -> w126
                      frame False {
                      }
                      frame True {
                        n341 = Bundle By Name(cluster=w143, "METHOD"=u16 1) -> (w141:T6)
                        n342 = call "VNARP-Detect resonance.vi"("RP VNA SETTING"=w139, "VNA DATA CLUSTER"=w140, "RESONNANCE DETECTION"=w141) -> ("Parabolic fit"=w138:cluster{cluster{dbl, dbl}[]})  [unwired: 6 in, 2 out]
                        n343 = Insert Into Array(array=w137, new element=w138) -> (w136:T14)  [unwired: 1 in]
                      }
                    }
                    n344 = property on="MAGNITUDE/PHASE" class="XYGraph (strict)"("Val(Sgnl)"=w126) -> ()  [unwired: 2 in, 2 out]
                  }
                  frame #2 {
                    n345 = local read "LOOP ACT"() -> (w147:bool)
                    n346 = Select(t="VNA LOOP" ("element"), s=w147, f="WAIT" ("element")) -> (s? t:f=w146:string)
                    n347 = Enqueue Element(queue=w148, element=w146) -> ()  [unwired: 2 in, 3 out]
                    n348 = stacked-sequence {
                      frame #0 {
                        n349 = local write "ACQ Indicator"(TRUE ("ACQ Indicator")) -> ()
                      }
                      frame #1 {
                        n350 = Wait (ms)(milliseconds to wait=u32 100 ("attente (ms)")) -> ()  [unwired: 1 out]
                      }
                      frame #2 {
                        n351 = local write "ACQ Indicator"(FALSE ("ACQ Indicator")) -> ()
                      }
                    }
                  }
                }
                n352 = Wait (ms)(milliseconds to wait=u32 10 ("attente (ms)")) -> ()  [unwired: 1 out]
              }
              frame "TRACK OBS" {
                n353 = local write "STATUS"(w157) -> ()
                n354 = stacked-sequence {
                  tunnel: w154 -> [w169 _ _ _]
                  tunnel: w153 -> [w168 _ _ _]
                  tunnel: w152 -> [_ _ _ w212]
                  frame #0 {
                    n355 = local read "SPECTRUM POST PROCESSING PARAMETERS"() -> (w165:cluster{"N° SMOOTHING POINTS":i32})
                    n356 = local read "RP VNA SETTING"() -> (w178:T1)
                    n357 = Unbundle By Name(w165) -> ("N° SMOOTHING POINTS"=w162:i32)
                    n358 = Unbundle By Name(w178) -> ("Sweep size"=w177:u32)
                    n359 = local read "RAW Freq table"() -> (w163:dbl[])
                    n360 = call "VNARP-CASES.vi"("entrée d'erreur (pas d'erreur)"=w168, "Setting"=u32 0, "Énum"=T11."SWEEP START", "ID de connexion"=w169) -> ("sortie d'erreur"=w176:errorcluster, "ID de connexion en sortie"=w179:refnum<k5>)  [unwired: 3 in]
                    n361 = call "VNARP-Read.vi"("SIZE"=w177, "entrée d'erreur (pas d'erreur)"=w176, "smoothing points"=w162, "Freq table IN"=w163, "ID de connexion"=w179) -> ("DATA OUT"=w161:T13)  [unwired: 4 in, 2 out]
                    n362 = Unbundle By Name(w161) -> ("FREQUENCY"=w159:sgl[], "MAGNITUDE 1"=w160:dbl[], "PHASE 1"=w158:dbl[])
                    n363 = local read "VNA DATA CLUSTER"() -> (w167:T9)
                    n364 = Build Cluster Array(w159, w158) -> (w174:cluster{sgl, dbl}[])
                    n365 = Build Cluster Array(w159, w158) -> (w175:cluster{sgl, dbl}[])
                    n366 = Bundle By Name(cluster=w167, "FREQUENCY TABLE"=w159, "MAGNITUDE TABLE"=w160, "PHASE TABLE"=w158) -> (w166:T9)
                    n367 = Bundle(w174) -> (w173:cluster{cluster{sgl, dbl}[]})  [unwired: 1 in]
                    n368 = Bundle(w175) -> (w172:cluster{cluster{sgl, dbl}[]})  [unwired: 1 in]
                    n369 = Build Array(w173, w172) -> (w164:cluster{cluster{sgl, dbl}[]}[])
                    n370 = local write "MAGNITUDE/PHASE"(w164) -> ()
                    n371 = property on="MAGNITUDE/PHASE" class="XYGraph (strict)"("Val(Sgnl)"=w164) -> ()  [unwired: 2 in, 2 out]
                    n372 = local write "VNA DATA CLUSTER"(w166) -> ()
                  }
                  frame #1 {
                    n373 = local read "RP VNA SETTING"() -> (w190:T1)
                    n374 = local read "VNA DATA CLUSTER"() -> (w192:T9)
                    n375 = Unbundle By Name(w190) -> ("Sweep size"=w189:u32)
                    n376 = Max & Min(x=500 ("Fit length"), y=w189) -> (min(x,y)=w187:u32)  [unwired: 1 out]
                    n377 = Unbundle By Name(w192) -> ("FREQUENCY TABLE"=w186:ext[], "MAGNITUDE TABLE"=w185:ext[])
                    n378 = call "VNARP PARABOLA FIT.vi"("Freq Table IN"=w186, "Fit length"=w187, "Y IN"=w185) -> ("Parabol max position"=w180:dbl)  [unwired: 3 out]
                    n379 = feedback #2() -> (w191:dbl[])
                    n380 = Build Array (concatenate)(w191, w180) -> (w183:dbl[])
                    n381 = call "Search Unsorted 1D Array.vim"("element"=0.0, "unsorted 1D array"=w183) -> ("index of element"=w184:i32)  [unwired: 9 in]
                    n382 = Delete From Array(array=w183, index=w184) -> (array with subset deleted=w181:dbl[])  [unwired: 1 in, 1 out]
                    n383 = feedback-in #2(w181) -> ()
                    n384 = local write "track data"(w181) -> ()
                  }
                  frame #2 {
                    n385 = local read "TEMPORAL SMOOTHING"() -> (w195:i32)
                    n386 = local read "track data"() -> (w193:dbl[])
                    n387 = Array Size(array=w193) -> (size(s)=w197:i32)
                    n388 = Subtract(x=w197, y=w195) -> (x-y=w198:i32)
                    n389 = for {
                      N: w198 -> [_]
                      tunnel: w195 -> [w206]
                      tunnel: w193 -> [w207]
                      tunnel: [w203] -> w196 mode=indexing
                      i -> [w205]
                      n390 = Array Subset(array=w207, index=w205, length=w206) -> (w204:dbl[])
                      n391 = call-poly <vilib>:"Mean.vi"("X"=w204) -> ("mean"=w203:dbl)  [unwired: 1 out]
                    }
                    n392 = local read "N°POINTS TO DISPLAY"() -> (w199:i32)
                    n393 = Array Size(array=w196) -> (size(s)=w201:i32)
                    n394 = Subtract(x=w201, y=w199) -> (x-y=w200:i32)
                    n395 = Max & Min(x=0.0, y=w200) -> (max(x,y)=w202:dbl)  [unwired: 1 out]
                    n396 = Array Subset(array=w196, index=w202, length=w199) -> ()  [unwired: 1 out]
                  }
                  frame #3 {
                    n397 = local read "LOOP ACT"() -> (w211:bool)
                    n398 = Select(t="TRACK" ("element"), s=w211, f="WAIT" ("element")) -> (s? t:f=w210:string)
                    n399 = Enqueue Element(queue=w212, element=w210) -> ()  [unwired: 2 in, 3 out]
                  }
                }
                n400 = Wait (ms)(milliseconds to wait=u32 10 ("attente (ms)")) -> ()  [unwired: 1 out]
              }
              frame "TRACK" {
                n401 = local write "STATUS"(w217) -> ()
                n402 = stacked-sequence {
                  tunnel: w215 -> [_ w224 _]
                  tunnel: w214 -> [_ w223 _]
                  tunnel: w213 -> [_ w222 w433]
                  frame #0 {
                    n403 = local read "DELAY BETWEEN TRIG (s)"() -> (w220:i32)
                    n404 = Multiply(x=w220, y=u32 1000 ("attente (ms)")) -> (x*y=w219:u32)
                    n405 = Wait (ms)(milliseconds to wait=w219) -> ()  [unwired: 1 out]
                  }
                  frame #1 {
                    n406 = local read "CHANNELS PARAMETERS"() -> (w221:T4[])
                    n407 = for {
                      tunnel: w221 -> [w230] mode=indexing
                      tunnel: w224 -> [w229]
                      tunnel: w223 -> [w228]
                      tunnel: w222 -> [w226]
                      tunnel: w221 -> [w225]
                      i -> [w227]
                      n408 = Unbundle By Name(w230) -> ("CHANNEL TRACK ?"=w231:bool)
                      n409 = case shown="True" w231 {
                        tunnel: w230 -> [_ w233]
                        tunnel: w229 -> [_ w234]
                        tunnel: w228 -> [_ w236]
                        tunnel: w227 -> [_ w235]
                        tunnel: w226 -> [_ _]
                        tunnel: w225 -> [_ w232]
                        frame False {
                        }
                        frame True {
                          n410 = stacked-sequence {
                            tunnel: w236 -> [_ w248 _ _ _ w277 w304 _ _ _ _ _ _ _ _]
                            tunnel: w235 -> [w237 _ _ _ w268 _ _ _ w319 w324 w343 _ _ _ _]
                            tunnel: w234 -> [_ w239 _ _ _ w274 w302 _ _ _ _ _ _ _ _]
                            tunnel: w233 -> [_ w238 _ _ w269 _ _ _ _ _ _ _ _ _ _]
                            tunnel: w232 -> [_ _ _ _ w267 _ _ _ _ _ _ _ _ _ _]
                            frame #0 {
                              # "ATTENTION : do not trig channel choice change event !!!!"
                              # "switch"
                              n411 = local write "CHANNEL CHOICE VNA"(w237) -> ()
                              n412 = local write "CHANNELS IND TRACK"(w237) -> ()
                            }
                            frame #1 {
                              n413 = local write "VNA SETTING CLUSTER"(w238) -> ()
                              n414 = local read "RP VNA SETTING"() -> (w251:T1)
                              n415 = call "VNARP-VNASETTING CLTR MANAGMENT.vi"("VNA SETTING CLUSTER"=w238, "RP VNA SETTING"=w251) -> ("OUTPUT VNA SETTINGS"=w249:T15)  [unwired: 1 in]
                              n416 = local write "RP VNA SETTING"(w249) -> ()
                              n417 = call "VNARP-SettingsUpdate.vi"("Error IN"=w248, "RP VNA SETTINGS IN"=w249, "ID de connexion IN"=w239) -> ("Freq table"=w250:dbl[])  [unwired: 2 out]
                              n418 = local write "RAW Freq table"(w250) -> ()
                              n419 = Unbundle By Name(w238) -> ("START 2"=w241:dbl, "STOP 2"=w247:dbl, "CENTER 2"=w246:dbl, "SPAN 2"=w245:dbl, "PUMP"=w240:dbl, "PROBE"=w244:dbl, "Points N° 2"=w243:i32, "SPACING 2"=w242:dbl)
                              n420 = local write "Points N°"(w243) -> ()
                              n421 = local write "SPACING"(w242) -> ()
                              n422 = local write "CENTER"(w246) -> ()
                              n423 = local write "START"(w241) -> ()
                              n424 = local write "STOP"(w247) -> ()
                              n425 = local write "PROBE"(w244) -> ()
                              n426 = local write "SPAN"(w245) -> ()
                              n427 = local write "PUMP"(w240) -> ()
                              n428 = property on="START" class="DigNum (strict)"("Val(Sgnl)"=w241) -> ()  [unwired: 2 in, 2 out]
                              n429 = property on="PUMP" class="Slide (strict)"("Val(Sgnl)"=w240) -> ()  [unwired: 2 in, 2 out]
                            }
                            frame #2 {
                              w260 = u16 0 items=["AOUT0", "AOUT1", "AOUT2", "AOUT3"] ("Pin #")
                              w259 = u16 1 items=["AOUT0", "AOUT1", "AOUT2", "AOUT3"] ("Pin #")
                              n430 = local read "VOA Calibration cluster"() -> (w258:cluster{"PUMP":dbl[], "PROBE":dbl[]})
                              n431 = local read "NETWORK PARAMETERS"() -> (w262:T8)
                              n432 = Unbundle By Name(w262) -> ("RP-IP 2"=w261:string)
                              n433 = Unbundle By Name(w258) -> ("PUMP"=w253:dbl[], "PROBE"=w256:dbl[])
                              n434 = local read "PUMP"() -> (w254:dbl)
                              n435 = local read "PROBE"() -> (w257:dbl)
                              n436 = call "RP-VOA CONVERSION P to V.vi"("Calibration points"=w253, "% power"=w254) -> ("DAC Voltage"=w252:dbl)
                              n437 = call "RP-VOA CONVERSION P to V.vi"("Calibration points"=w256, "% power"=w257) -> ("DAC Voltage"=w255:dbl)
                              n438 = call "RP-ANALOG-OUT.vi"("Voltage"=w252, "Pin #"=w260, "IP address"=w261) -> ()  [unwired: 1 out]
                              n439 = call "RP-ANALOG-OUT.vi"("Voltage"=w255, "Pin #"=w259, "IP address"=w261) -> ()  [unwired: 1 out]
                            }
                            frame #3 {
                              n440 = local read "VNA SETTING CLUSTER"() -> (w266:T4)
                              n441 = local read "PROBE"() -> (w264:dbl)
                              n442 = local read "PUMP"() -> (w265:dbl)
                              n443 = Bundle By Name(cluster=w266, "PUMP"=w265, "PROBE"=w264) -> (w263:T4)
                              n444 = local write "VNA SETTING CLUSTER"(w263) -> ()
                            }
                            frame #4 {
                              n445 = local read "VNA SETTING CLUSTER"() -> (w272:T4)
                              n446 = Unbundle By Name(w269) -> ("CHANNEL TRACK ?"=w271:bool)
                              n447 = Bundle By Name(cluster=w272, "CHANNEL TRACK ?"=w271) -> (w270:T4)
                              n448 = Replace Array Subset(array=w267, new element=w270, index=w268) -> (w273:T4[])
                              n449 = local write "CHANNELS PARAMETERS"(w273) -> ()
                            }
                            frame #5 {
                              # "wait for stab"
                              n450 = local read "DELAY AFTER SWITCH (s)"() -> (w276:i32)
                              n451 = Equal To 0?(x=w276) -> (x = 0?=w275:bool)
                              n452 = case shown="False" w275 {
                                tunnel: w277 -> [w279 _]
                                tunnel: w274 -> [w278 _]
                                frame False {
                                n453 = Tick Count (ms)() -> (millisecond timer value=w280:u32)
                                n454 = while {
                                tunnel: w280 -> [w289]
                                tunnel: w279 -> [w283]
                                tunnel: w278 -> [w282]
                                stop <- w284 stop-if-true
                                n455 = flat-sequence {
                                tunnel: w283 -> [_]
                                tunnel: w282 -> [_]
                                tunnel: [w290] -> w281
                                frame #0 {
                                }
                                frame #1 {
                                n456 = Tick Count (ms)() -> (millisecond timer value=w290:u32)
                                }
                                }
                                n457 = local read "DELAY AFTER SWITCH (s)"() -> (w288:i32)
                                n458 = Subtract(x=w281, y=w289) -> (x-y=w286:u32)
                                n459 = Multiply(x=w288, y=1000) -> (x*y=w285:i32)
                                n460 = Greater Or Equal?(x=w286, y=w285) -> (x >= y?=w284:bool)
                                }
                                }
                                frame True {
                                }
                              }
                            }
                            frame #6 {
                              # "AVERAGING IS MISSING !"
                              n461 = local read "SPECTRUM POST PROCESSING PARAMETERS"() -> (w307:cluster{"N° SMOOTHING POINTS":i32})
                              n462 = Unbundle By Name(w307) -> ("N° SMOOTHING POINTS"=w298:i32)
                              n463 = local read "RP VNA SETTING"() -> (w310:T1)
                              n464 = local read "RAW Freq table"() -> (w297:dbl[])
                              n465 = Unbundle By Name(w310) -> ("Sweep size"=w299:u32)
                              n466 = call "VNARP-CASES.vi"("entrée d'erreur (pas d'erreur)"=w304, "Setting"=u32 0, "Énum"=T11."SWEEP START", "ID de connexion"=w302) -> ("sortie d'erreur"=w300:errorcluster, "ID de connexion en sortie"=w301:refnum<k5>)  [unwired: 3 in]
                              n467 = local read "CHANNEL CHOICE VNA"() -> (w303:T3)
                              n468 = call "VNARP-Read.vi"("SIZE"=w299, "entrée d'erreur (pas d'erreur)"=w300, "smoothing points"=w298, "Freq table IN"=w297, "ID de connexion"=w301) -> ("DATA OUT"=w296:T13)  [unwired: 4 in, 2 out]
                              n469 = Unbundle By Name(w296) -> ("FREQUENCY"=w295:sgl[], "REAL 1"=w294:dbl[], "IMAGINARY 1"=w293:sgl[], "MAGNITUDE 1"=w292:dbl[], "PHASE 1"=w291:dbl[])
                              n470 = local read "VNA DATA CLUSTER"() -> (w309:T9)
                              n471 = Bundle By Name(cluster=w309, "CHANNEL"=w303, "FREQUENCY TABLE"=w295, "REAL TABLE"=w294, "IMAGINARY TABLE"=w293, "MAGNITUDE TABLE"=w292, "PHASE TABLE"=w291) -> (w308:T9)
                              n472 = local write "VNA DATA CLUSTER"(w308) -> ()
                            }
                            frame #7 {
                              n473 = local read "PERSISTANCE DATA CLUSTER"() -> (w313:T9)
                              n474 = local read "VNA DATA CLUSTER"() -> (w314:T9)
                              n475 = local read "BTN DISPLAY TYPE"() -> (w315:bool)
                              n476 = local read "BTN VIEW PERSISTANCE"() -> (w312:bool)
                              n477 = call "MAKE DISPLAY ARRAY.vi"("VNA DATA CLUSTER"=w314, "PERSISTANCE DATA CLUSTER"=w313, "Display type (F : MAG/PHASE)"=w315, "Persistance"=w312) -> ("Display array"=w311:T14)  [unwired: 2 in]
                              n478 = local write "MAGNITUDE/PHASE"(w311) -> ()
                              n479 = property on="MAGNITUDE/PHASE" class="XYGraph (strict)"("Val(Sgnl)"=w311) -> ()  [unwired: 2 in, 2 out]
                              n480 = stacked-sequence {
                                frame #0 {
                                n481 = local write "ACQ Indicator"(TRUE ("ACQ Indicator")) -> ()
                                }
                                frame #1 {
                                n482 = Wait (ms)(milliseconds to wait=u32 100) -> ()  [unwired: 1 out]
                                }
                                frame #2 {
                                n483 = local write "ACQ Indicator"(FALSE ("ACQ Indicator")) -> ()
                                }
                              }
                            }
                            frame #8 {
                              n484 = local read "VNA DATA CLUSTER TBL"() -> (w321:T9[])
                              n485 = local read "VNA DATA CLUSTER"() -> (w320:T9)
                              n486 = Replace Array Subset(array=w321, new element=w320, index=w319) -> (w322:T9[])
                              n487 = local write "VNA DATA CLUSTER TBL"(w322) -> ()
                            }
                            frame #9 {
                              n488 = local read "BTN AUTOSAVE RAW DATA"() -> (w323:bool)
                              n489 = case shown="True" w323 {
                                tunnel: w324 -> [_ w326]
                                frame False {
                                }
                                frame True {
                                # "save to file vna"
                                n490 = local read "VNA DATA CLUSTER TBL"() -> (w337:T9[])
                                n491 = local read "Track Repositery List"() -> (w327:path[])
                                n492 = Tick Count (ms)() -> (millisecond timer value=w335:u32)
                                n493 = Number To Decimal String(number=w335) -> (decimal integer string=w334:string)  [unwired: 1 in]
                                n494 = call "RP-VNA DATA TBL Extract.vi"("VNA DATA CLUSTER TBL"=w337, "index"=w326) -> ("appended array"=w336:ext[][])  [unwired: 2 in, 1 out]
                                n495 = Concatenate Strings("RAW VNA DATA " ("string"), w334, ".txt" ("string")) -> (w332:string)
                                n496 = Index Array(array=w327, index=w326) -> (element=w325:path)
                                n497 = Build Path(base path=w325, name or relative path=w332) -> (appended path=w331:path)
                                n498 = call-poly <vilib>:"Write Delimited Spreadsheet.vi"("file path (dialog if empty)"=w331, "format (%.3f)"="%.6f", "2D data"=w336, "transpose? (no:F)"=TRUE) -> ()  [unwired: 10 in, 2 out]
                                }
                              }
                            }
                            frame #10 {
                              # "add to track kpi tables"
                              n499 = local read "RESONNANCE DETECTION"() -> (w340:T6)
                              n500 = local read "VNA DATA CLUSTER"() -> (w339:T9)
                              n501 = local read "RP VNA SETTING"() -> (w338:T1)
                              n502 = local read "TRACK DATA CLUSTER TBL"() -> (w345:cluster{"CHANNEL":dbl, "KPI 1 TRACK":ext[]}[])
                              n503 = local read "BTN FIT DISPLAY"() -> (w341:bool)
                              n504 = call "VNARP-Detect resonance.vi"("RP VNA SETTING"=w338, "VNA DATA CLUSTER"=w339, "RESONNANCE DETECTION"=w340) -> ("Resonant frequency"=w342:ext)  [unwired: 6 in, 2 out]
                              n505 = Index Array(array=w345, index=w343) -> (element=w347:cluster{"CHANNEL":dbl, "KPI 1 TRACK":ext[]})
                              n506 = Unbundle By Name(w347) -> ("KPI 1 TRACK"=w349:ext[])
                              n507 = case shown="True" w341 {
                                tunnel: w340 -> [_ w355]
                                tunnel: w339 -> [_ w352]
                                tunnel: w338 -> [_ w351]
                                frame False {
                                }
                                frame True {
                                n508 = Bundle By Name(cluster=w355, "METHOD"=u16 1) -> (w353:T6)
                                n509 = property on="MAGNITUDE/PHASE" class="XYGraph (strict)"() -> ("Value"=w357:cluster{cluster{dbl, dbl}[]}[])  [unwired: 2 in, 2 out]
                                n510 = call "VNARP-Detect resonance.vi"("RP VNA SETTING"=w351, "VNA DATA CLUSTER"=w352, "RESONNANCE DETECTION"=w353) -> ("Parabolic fit"=w350:cluster{cluster{dbl, dbl}[]})  [unwired: 6 in, 2 out]
                                n511 = Insert Into Array(array=w357, new element=w350) -> (w356:cluster{cluster{dbl, dbl}[]}[])  [unwired: 1 in]
                                n512 = property on="MAGNITUDE/PHASE" class="XYGraph (strict)"("Val(Sgnl)"=w356) -> ()  [unwired: 2 in, 2 out]
                                }
                              }
                              n513 = Build Array (concatenate)(w349, w342) -> (w348:ext[])
                              n514 = Bundle By Name(cluster=w347, "CHANNEL"=w343, "KPI 1 TRACK"=w348) -> (w346:cluster{"CHANNEL":dbl, "KPI 1 TRACK":ext[]})
                              n515 = Replace Array Subset(array=w345, new element=w346, index=w343) -> (w344:cluster{"CHANNEL":dbl, "KPI 1 TRACK":ext[]}[])
                              n516 = local write "TRACK DATA CLUSTER TBL"(w344) -> ()
                            }
                            frame #11 {
                              n517 = local read "TRACK DATA CLUSTER TBL"() -> (w361:cluster{"CHANNEL":dbl, "KPI 1 TRACK":ext[]}[])
                              n518 = for {
                                tunnel: w361 -> [w386] mode=indexing
                                tunnel: [w364] -> w360 mode=indexing
                                tunnel: [w363] -> w359 mode=indexing
                                tunnel: [w362] -> w358 mode=indexing
                                n519 = local read "TEMPORAL SMOOTHING"() -> (w383:i32)
                                n520 = Unbundle By Name(w386) -> ("KPI 1 TRACK"=w382:ext[])
                                n521 = Array Size(array=w382) -> (size(s)=w384:i32)
                                n522 = Subtract(x=w384, y=w383) -> (x-y=w385:i32)
                                n523 = for {
                                N: w385 -> [_]
                                tunnel: w383 -> [w390]
                                tunnel: w382 -> [w391]
                                tunnel: [w387] -> w371 mode=indexing
                                i -> [w389]
                                n524 = Array Subset(array=w391, index=w389, length=w390) -> (w388:ext[])
                                n525 = call-poly <vilib>:"Mean.vi"("X"=w388) -> ("mean"=w387:dbl)  [unwired: 1 out]
                                }
                                n526 = Delete From Array(array=w371, length=1, index=0) -> (array with subset deleted=w363:dbl[])  [unwired: 1 out]
                                n527 = local read "DISPLAY OPTION"() -> (w380:u16)
                                n528 = Index Array(array=w363, index=0) -> (element=w375:dbl)
                                n529 = local read "N°POINTS TO DISPLAY"() -> (w367:i32)
                                n530 = Subtract(x=w363, y=w375) -> (x-y=w376:dbl[])
                                n531 = Divide(x=w376, y=w375) -> (x/y=w374:dbl[])
                                n532 = Equal?(x=w380, y=u16 0) -> (x = y?=w372:bool)
                                n533 = Multiply(x=w374, y=1000000.0 ("f")) -> (x*y=w362:dbl[])
                                n534 = Select(t=w363, s=w372, f=w362) -> (s? t:f=w365:dbl[])
                                n535 = Array Size(array=w365) -> (size(s)=w369:i32)
                                n536 = Subtract(x=w369, y=w367) -> (x-y=w368:i32)
                                n537 = Max & Min(x=0.0, y=w368) -> (max(x,y)=w370:dbl)  [unwired: 1 out]
                                n538 = Array Subset(array=w365, index=w370) -> (w364:dbl[])  [unwired: 1 in]
                              }
                              n539 = local write "TRACK DATA ABS"(w359) -> ()
                              n540 = local write "TRACK DATA REL"(w358) -> ()
                              n541 = local write "LIVE TRACK"(w360) -> ()
                            }
                            frame #12 {
                              n542 = local read "TRACK DATA CLUSTER TBL"() -> (w394:cluster{"CHANNEL":dbl, "KPI 1 TRACK":ext[]}[])
                              n543 = for {
                                tunnel: w394 -> [w407] mode=indexing
                                tunnel: [w398] -> w393 mode=indexing
                                tunnel: [w397] -> w392 mode=indexing
                                n544 = Unbundle By Name(w407) -> ("KPI 1 TRACK"=w396:ext[])
                                n545 = local read "DISPLAY OPTION"() -> (w405:u16)
                                n546 = Delete From Array(array=w396, length=1, index=0) -> (array with subset deleted=w398:ext[])  [unwired: 1 out]
                                n547 = Equal?(x=w405, y=u16 0) -> ()  [unwired: 1 out]
                                n548 = Index Array(array=w398, index=0) -> (element=w400:ext)
                                n549 = Subtract(x=w398, y=w400) -> (x-y=w401:ext[])
                                n550 = Divide(x=w401, y=w400) -> (x/y=w399:ext[])
                                n551 = Multiply(x=w399, y=1000000.0 ("f")) -> (x*y=w397:ext[])
                              }
                              n552 = local write "TRACK DATA ABS NO SMOOTHING"(w393) -> ()
                              n553 = local write "TRACK DATA REL NO SMOOTHING"(w392) -> ()
                            }
                            frame #13 {
                              n554 = local read "TRACK DATA ABS NO SMOOTHING"() -> (w416:dbl[][])
                              n555 = local read "TRACK REPOSITERY"() -> (w429:path)
                              n556 = local read "TRACK REPOSITERY"() -> (w410:path)
                              n557 = local read "TRACK DATA ABS"() -> (w423:dbl[][])
                              n558 = Build Path(base path=w429, name or relative path="ALL CHANNEL ABS Track.txt") -> (appended path=w430:path)
                              n559 = Build Path(base path=w410, name or relative path="ALL CHANNEL ABS Track NS.txt") -> (appended path=w409:path)
                              n560 = call-poly <vilib>:"Write Delimited Spreadsheet.vi"("file path (dialog if empty)"=w430, "format (%.3f)"="%.6f", "2D data"=w423, "transpose? (no:F)"=TRUE) -> ()  [unwired: 10 in, 2 out]
                              n561 = call-poly <vilib>:"Write Delimited Spreadsheet.vi"("file path (dialog if empty)"=w409, "format (%.3f)"="%.6f", "2D data"=w416, "transpose? (no:F)"=TRUE) -> ()  [unwired: 10 in, 2 out]
                              n562 = local read "TRACK DATA REL NO SMOOTHING"() -> (w417:dbl[][])
                              n563 = local read "TRACK REPOSITERY"() -> (w426:path)
                              n564 = local read "TRACK REPOSITERY"() -> (w413:path)
                              n565 = local read "TRACK DATA REL"() -> (w422:dbl[][])
                              n566 = Build Path(base path=w426, name or relative path="ALL CHANNEL REL Track.txt") -> (appended path=w425:path)
                              n567 = Build Path(base path=w413, name or relative path="ALL CHANNEL REL Track NS.txt") -> (appended path=w414:path)
                              n568 = call-poly <vilib>:"Write Delimited Spreadsheet.vi"("file path (dialog if empty)"=w425, "format (%.3f)"="%.6f", "2D data"=w422, "transpose? (no:F)"=TRUE) -> ()  [unwired: 10 in, 2 out]
                              n569 = call-poly <vilib>:"Write Delimited Spreadsheet.vi"("file path (dialog if empty)"=w414, "format (%.3f)"="%.6f", "2D data"=w417, "transpose? (no:F)"=TRUE) -> ()  [unwired: 10 in, 2 out]
                            }
                            frame #14 {
                            }
                          }
                        }
                      }
                    }
                  }
                  frame #2 {
                    n570 = local read "LOOP ACT"() -> (w436:bool)
                    n571 = Select(t="TRACK" ("element"), s=w436, f="WAIT" ("element")) -> (s? t:f=w435:string)
                    n572 = Enqueue Element(queue=w433, element=w435) -> ()  [unwired: 2 in, 3 out]
                  }
                }
              }
              frame "RUN VNA" {
                n573 = local write "STATUS"(w441) -> ()
                n574 = stacked-sequence {
                  tunnel: w439 -> [w460 _ _]
                  tunnel: w438 -> [w459 _ _]
                  frame #0 {
                    n575 = local read "RP VNA SETTING"() -> (w455:T1)
                    n576 = local read "SPECTRUM POST PROCESSING PARAMETERS"() -> (w450:cluster{"N° SMOOTHING POINTS":i32})
                    n577 = Unbundle By Name(w450) -> ("N° SMOOTHING POINTS"=w448:i32)
                    n578 = local read "RAW Freq table"() -> (w449:dbl[])
                    n579 = Unbundle By Name(w455) -> ("Sweep size"=w454:u32)
                    n580 = call "VNARP-CASES.vi"("entrée d'erreur (pas d'erreur)"=w459, "Setting"=u32 0, "Énum"=T11."SWEEP START", "ID de connexion"=w460) -> ("sortie d'erreur"=w453:errorcluster, "ID de connexion en sortie"=w456:refnum<k5>)  [unwired: 3 in]
                    n581 = local read "VNA DATA CLUSTER"() -> (w452:T9)
                    n582 = call "VNARP-Read.vi"("SIZE"=w454, "entrée d'erreur (pas d'erreur)"=w453, "smoothing points"=w448, "Freq table IN"=w449, "ID de connexion"=w456) -> ("DATA OUT"=w447:T13)  [unwired: 4 in, 2 out]
                    n583 = Unbundle By Name(w447) -> ("FREQUENCY"=w446:sgl[], "MAGNITUDE 1"=w445:dbl[], "PHASE 1"=w444:dbl[], "REAL 1"=w443:dbl[], "IMAGINARY 1"=w442:sgl[])
                    n584 = Bundle By Name(cluster=w452, "FREQUENCY TABLE"=w446, "MAGNITUDE TABLE"=w445, "PHASE TABLE"=w444, "REAL TABLE"=w443, "IMAGINARY TABLE"=w442) -> (w451:T9)
                    n585 = local write "VNA DATA CLUSTER"(w451) -> ()
                  }
                  frame #1 {
                    n586 = local read "VNA DATA CLUSTER"() -> (w465:T9)
                    n587 = local read "PERSISTANCE DATA CLUSTER"() -> (w468:T9)
                    n588 = local read "BTN DISPLAY TYPE"() -> (w469:bool)
                    n589 = local read "BTN VIEW PERSISTANCE"() -> (w467:bool)
                    n590 = local read "RESONNANCE DETECTION"() -> (w462:T6)
                    n591 = local read "RP VNA SETTING"() -> (w463:T1)
                    n592 = local read "BTN FIT DISPLAY"() -> (w464:bool)
                    n593 = call "MAKE DISPLAY ARRAY.vi"("VNA DATA CLUSTER"=w465, "PERSISTANCE DATA CLUSTER"=w468, "Display type (F : MAG/PHASE)"=w469, "Persistance"=w467) -> ("Display array"=w466:T14)  [unwired: 2 in]
                    n594 = case shown="True" w464 {
                      tunnel: w462 -> [_ w478]
                      tunnel: w465 -> [_ w475]
                      tunnel: w463 -> [_ w474]
                      tunnel: w466 -> [w470 w472]
                      tunnel: [w470 w471] -> w461
                      frame False {
                      }
                      frame True {
                        n595 = Bundle By Name(cluster=w478, "METHOD"=u16 1) -> (w476:T6)
                        n596 = call "VNARP-Detect resonance.vi"("RP VNA SETTING"=w474, "VNA DATA CLUSTER"=w475, "RESONNANCE DETECTION"=w476) -> ("Parabolic fit"=w473:cluster{cluster{dbl, dbl}[]})  [unwired: 6 in, 2 out]
                        n597 = Insert Into Array(array=w472, new element=w473) -> (w471:T14)  [unwired: 1 in]
                      }
                    }
                    n598 = property on="MAGNITUDE/PHASE" class="XYGraph (strict)"("Val(Sgnl)"=w461) -> ()  [unwired: 2 in, 2 out]
                  }
                  frame #2 {
                    n599 = stacked-sequence {
                      frame #0 {
                        n600 = local write "ACQ Indicator"(TRUE ("ACQ Indicator")) -> ()
                      }
                      frame #1 {
                        n601 = Wait (ms)(milliseconds to wait=u32 100 ("attente (ms)")) -> ()  [unwired: 1 out]
                      }
                      frame #2 {
                        n602 = local write "ACQ Indicator"(FALSE ("ACQ Indicator")) -> ()
                      }
                    }
                  }
                }
                n603 = Wait (ms)(milliseconds to wait=u32 10 ("attente (ms)")) -> ()  [unwired: 1 out]
              }
              frame "CHANNEL CHANGE" {
                n604 = stacked-sequence {
                  frame #0 {
                    n605 = local read "CHANNEL CHOICE VNA"() -> (w494:T3)
                    n606 = local read "CHANNELS PARAMETERS"() -> (w495:T4[])
                    n607 = Index Array(array=w495, index=w494) -> (element=w491:T4)
                    n608 = local write "VNA SETTING CLUSTER"(w491) -> ()
                    n609 = local read "RP VNA SETTING"() -> (w492:T1)
                    n610 = Unbundle By Name(w491) -> ("START 2"=w485:dbl, "STOP 2"=w490:dbl, "CENTER 2"=w489:dbl, "SPAN 2"=w488:dbl, "PUMP"=w483:dbl, "PROBE"=w484:dbl, "Points N° 2"=w487:i32, "SPACING 2"=w486:dbl)
                    n611 = local write "Points N°"(w487) -> ()
                    n612 = local write "SPACING"(w486) -> ()
                    n613 = local write "CENTER"(w489) -> ()
                    n614 = local write "START"(w485) -> ()
                    n615 = local write "STOP"(w490) -> ()
                    n616 = local write "PROBE"(w484) -> ()
                    n617 = local write "SPAN"(w488) -> ()
                    n618 = local write "PUMP"(w483) -> ()
                    n619 = call "VNARP-VNASETTING CLTR MANAGMENT.vi"("VNA SETTING CLUSTER"=w491, "RP VNA SETTING"=w492) -> ("OUTPUT VNA SETTINGS"=w493:T15)  [unwired: 1 in]
                    n620 = local write "RP VNA SETTING"(w493) -> ()
                    n621 = property on="START" class="DigNum (strict)"("Val(Sgnl)"=w485) -> ()  [unwired: 2 in, 2 out]
                  }
                  frame #1 {
                    w506 = u16 0 items=["AOUT0", "AOUT1", "AOUT2", "AOUT3"] ("Pin #")
                    w505 = u16 1 items=["AOUT0", "AOUT1", "AOUT2", "AOUT3"] ("Pin #")
                    n622 = local read "VOA Calibration cluster"() -> (w504:cluster{"PUMP":dbl[], "PROBE":dbl[]})
                    n623 = local read "NETWORK PARAMETERS"() -> (w507:T8)
                    n624 = local read "PROBE"() -> (w503:dbl)
                    n625 = Unbundle By Name(w507) -> ("RP-IP 2"=w497:string)
                    n626 = Unbundle By Name(w504) -> ("PUMP"=w498:dbl[], "PROBE"=w502:dbl[])
                    n627 = local read "PUMP"() -> (w499:dbl)
                    n628 = local read "CHANNEL CHOICE VNA"() -> (w496:T3)
                    n629 = call "RP-VOA CONVERSION P to V.vi"("Calibration points"=w498, "% power"=w499) -> ("DAC Voltage"=w500:dbl)
                    n630 = call "RP-VOA CONVERSION P to V.vi"("Calibration points"=w502, "% power"=w503) -> ("DAC Voltage"=w501:dbl)
                    n631 = call "RP-ANALOG-OUT.vi"("Voltage"=w500, "Pin #"=w506, "IP address"=w497) -> ()  [unwired: 1 out]
                    n632 = call "RP-ANALOG-OUT.vi"("Voltage"=w501, "Pin #"=w505, "IP address"=w497) -> ()  [unwired: 1 out]
                    n633 = call "RP-SWITCH CHANNEL.vi"("Channel"=w496, "IP address"=w497) -> ()  [unwired: 1 in, 1 out]
                  }
                  frame #2 {
                    n634 = local read "VNA SETTING CLUSTER"() -> (w511:T4)
                    n635 = local read "PROBE"() -> (w509:dbl)
                    n636 = local read "PUMP"() -> (w510:dbl)
                    n637 = Bundle By Name(cluster=w511, "PUMP"=w510, "PROBE"=w509) -> (w508:T4)
                    n638 = local write "VNA SETTING CLUSTER"(w508) -> ()
                  }
                  frame #3 {
                    n639 = local read "CHANNELS PARAMETERS"() -> (w517:T4[])
                    n640 = local read "CHANNEL CHOICE VNA"() -> (w516:T3)
                    n641 = Index Array(array=w517, index=w516) -> (element=w515:T4)
                    n642 = local read "VNA SETTING CLUSTER"() -> (w514:T4)
                    n643 = Unbundle By Name(w515) -> ("CHANNEL TRACK ?"=w513:bool)
                    n644 = Bundle By Name(cluster=w514, "CHANNEL TRACK ?"=w513) -> (w512:T4)
                    n645 = Replace Array Subset(array=w517, new element=w512, index=w516) -> (w518:T4[])
                    n646 = local write "CHANNELS PARAMETERS"(w518) -> ()
                  }
                  frame #4 {
                    n647 = local read "CHANNEL CHOICE VNA"() -> (→"CHANNEL CHOSEN":T3)
                  }
                }
              }
              frame "WAIT" {
                n648 = local write "STATUS"(w520) -> ()
              }
              frame "UPDATE" {
                n649 = local write "STATUS"(w525) -> ()
                n650 = stacked-sequence {
                  tunnel: w524 -> [w529 _ _]
                  tunnel: w523 -> [w527 _ _]
                  frame #0 {
                    n651 = local read "RP VNA SETTING"() -> (w528:T1)
                    n652 = call "VNARP-SettingsUpdate.vi"("Error IN"=w527, "RP VNA SETTINGS IN"=w528, "ID de connexion IN"=w529) -> ("Freq table"=w526:dbl[])  [unwired: 2 out]
                    n653 = local write "RAW Freq table"(w526) -> ()
                  }
                  frame #1 {
                    n654 = local read "VNA SETTING CLUSTER"() -> (w537:T4)
                    n655 = local read "Points N°"() -> (w531:i32)
                    n656 = local read "SPACING"() -> (w530:dbl)
                    n657 = local read "CENTER"() -> (w533:dbl)
                    n658 = local read "START"() -> (w536:dbl)
                    n659 = local read "SPAN"() -> (w532:dbl)
                    n660 = local read "STOP"() -> (w535:dbl)
                    n661 = Bundle By Name(cluster=w537, "START 2"=w536, "STOP 2"=w535, "CENTER 2"=w533, "SPAN 2"=w532, "Points N° 2"=w531, "SPACING 2"=w530) -> (w534:T4)
                    n662 = local write "VNA SETTING CLUSTER"(w534) -> ()
                  }
                  frame #2 {
                    n663 = local read "CHANNELS PARAMETERS"() -> (w543:T4[])
                    n664 = local read "CHANNEL CHOICE VNA"() -> (w542:T3)
                    n665 = Index Array(array=w543, index=w542) -> (element=w541:T4)
                    n666 = local read "VNA SETTING CLUSTER"() -> (w540:T4)
                    n667 = Unbundle By Name(w541) -> ("CHANNEL TRACK ?"=w539:bool)
                    n668 = Bundle By Name(cluster=w540, "CHANNEL TRACK ?"=w539) -> (w538:T4)
                    n669 = Replace Array Subset(array=w543, new element=w538, index=w542) -> (w544:T4[])
                    n670 = local write "CHANNELS PARAMETERS"(w544) -> ()
                  }
                }
              }
              frame "POWER UPDATE" {
                n671 = local write "STATUS"(w545) -> ()
                n672 = stacked-sequence {
                  frame #0 {
                    w555 = u16 0 items=["AOUT0", "AOUT1", "AOUT2", "AOUT3"] ("Pin #")
                    w557 = u16 1 items=["AOUT0", "AOUT1", "AOUT2", "AOUT3"] ("Pin #")
                    n673 = local read "VOA Calibration cluster"() -> (w553:cluster{"PUMP":dbl[], "PROBE":dbl[]})
                    n674 = local read "NETWORK PARAMETERS"() -> (w556:T8)
                    n675 = Unbundle By Name(w556) -> ("RP-IP 2"=w554:string)
                    n676 = Unbundle By Name(w553) -> ("PUMP"=w548:dbl[], "PROBE"=w551:dbl[])
                    n677 = local read "PUMP"() -> (w549:dbl)
                    n678 = local read "PROBE"() -> (w552:dbl)
                    n679 = call "RP-VOA CONVERSION P to V.vi"("Calibration points"=w548, "% power"=w549) -> ("DAC Voltage"=w547:dbl)
                    n680 = call "RP-VOA CONVERSION P to V.vi"("Calibration points"=w551, "% power"=w552) -> ("DAC Voltage"=w550:dbl)
                    n681 = call "RP-ANALOG-OUT.vi"("Voltage"=w550, "Pin #"=w557, "IP address"=w554) -> ()  [unwired: 1 out]
                    n682 = call "RP-ANALOG-OUT.vi"("Voltage"=w547, "Pin #"=w555, "IP address"=w554) -> ()  [unwired: 1 out]
                  }
                  frame #1 {
                    n683 = local read "VNA SETTING CLUSTER"() -> (w561:T4)
                    n684 = local read "PROBE"() -> (w559:dbl)
                    n685 = local read "PUMP"() -> (w560:dbl)
                    n686 = Bundle By Name(cluster=w561, "PUMP"=w560, "PROBE"=w559) -> (w558:T4)
                    n687 = local write "VNA SETTING CLUSTER"(w558) -> ()
                  }
                  frame #2 {
                    n688 = local read "CHANNELS PARAMETERS"() -> (w567:T4[])
                    n689 = local read "CHANNEL CHOICE VNA"() -> (w566:T3)
                    n690 = Index Array(array=w567, index=w566) -> (element=w565:T4)
                    n691 = local read "VNA SETTING CLUSTER"() -> (w564:T4)
                    n692 = Unbundle By Name(w565) -> ("CHANNEL TRACK ?"=w563:bool)
                    n693 = Bundle By Name(cluster=w564, "CHANNEL TRACK ?"=w563) -> (w562:T4)
                    n694 = Replace Array Subset(array=w567, new element=w562, index=w566) -> (w568:T4[])
                    n695 = local write "CHANNELS PARAMETERS"(w568) -> ()
                  }
                }
              }
              frame "SAVE VNA" {
                n696 = local read "TRACK DATA PARAMETERS"() -> (w576:cluster{"MAIN FOLDER":path})
                n697 = Unbundle By Name(w576) -> ("MAIN FOLDER"=w572:path)
                n698 = Build Path(base path=w572, name or relative path=path "SAVED VNA SPECTRUMS ") -> (appended path=w573:path)
                n699 = call <vilib>:"Check if File or Folder Exists.vi"("path"=w573) -> ("file or folder exists?"=w575:bool, "dup path"=w574:path)  [unwired: 8 in, 1 out]
                n700 = case shown="True" w575 {
                  tunnel: [w581 w582] -> w570
                  tunnel: w574 -> [w580 w582]
                  frame False {
                    n701 = Create Folder(path (use dialog)=w580) -> (created path=w581:path)  [unwired: 2 in, 2 out]
                  }
                  frame True {
                  }
                }
                n702 = call "File Dialog"("start path"=w570) -> ("selected path"=w577:path, "cancelled"=w578:bool, "error out"=w569:errorcluster)  [unwired: 11 in, 1 out]
                n703 = case shown="False" w578 {
                  tunnel: w577 -> [w585 _]
                  tunnel: w569 -> [_ _]
                  frame False {
                    n704 = local read "VNA DATA CLUSTER"() -> (w593:T9)
                    n705 = Unbundle By Name(w593) -> ("FREQUENCY TABLE"=w592:ext[], "MAGNITUDE TABLE"=w591:ext[], "PHASE TABLE"=w590:ext[], "REAL TABLE"=w584:ext[], "IMAGINARY TABLE"=w583:ext[])
                    n706 = Build Array(w592, w591, w590, w584, w583) -> (w588:ext[][])
                    n707 = call-poly <vilib>:"Write Delimited Spreadsheet.vi"("file path (dialog if empty)"=w585, "format (%.3f)"="%.6f", "2D data"=w588, "append to file? (new file:F)"=FALSE, "transpose? (no:F)"=TRUE) -> ()  [unwired: 9 in, 2 out]
                  }
                  frame True {
                  }
                }
              }
              frame "STOP" {
                w596 = FALSE ("TRACK-STOP")
                n708 = local write "STATUS"(w595) -> ()
                n709 = local read "RP CONNECT"() -> (w594:bool)
                n710 = case shown="True" w594 {
                  tunnel: w598 -> [_ w601]
                  tunnel: w597 -> [_ w600]
                  frame False {
                  }
                  frame True {
                    n711 = TCP Close Connection(connection ID=w601, error in (no error)=w600) -> ()  [unwired: 1 in, 2 out]
                  }
                }
                n712 = local write "TRACK-STOP"(w596) -> ()
                n713 = local write "LOOP ACT"(w596) -> ()
              }
            }
          }
          frame Error {
          }
        }
      }
      n714 = And(x=w71, y=w70) -> (x .and. y?=w69:bool)
      n715 = case shown="True" w69 {
        tunnel: w80 -> [_ w84]
        tunnel: w78 -> [_ w83]
        frame False {
        }
        frame True {
          n716 = Release Queue(queue=w83, error in (no error)=w84) -> ()  [unwired: 1 in, 3 out]
          n717 = property on="MAIN TAB" class="TabCtl (strict)"("Tabs Visible?"=TRUE ("Onglets visibles ?")) -> ()  [unwired: 2 in, 2 out]
        }
      }
    }
  }
